vi "main 1.2 dev.vi"() -> ()   [LabVIEW 2015]
uses:
  subvi/PHOIBOS/DEFINITIONS/DEF_dev_state.ctl
  subvi/PHOIBOS/DEFINITIONS/DEF_dev_type.ctl
  <vilib>/Analysis/6fits.llb/Curve Fitting Criteria.ctl
  <vilib>/Analysis/_algsub.llb/Real Vector Norm.vi
  <vilib>/Analysis/1siggen.llb/Ramp Pattern by Samples.vi
  <vilib>/DAQmx/create/channels.llb/DAQmx Create Channel (DI-Digital Input).vi
  <vilib>/Utility/file.llb/Write Delimited Spreadsheet (DBL).vi
  <vilib>/Utility/file.llb/Write Delimited Spreadsheet (string).vi
  <vilib>/Utility/file.llb/Read Delimited Spreadsheet (string).vi
  subvi/Newport ESP301/Newport ESP301.lvlib
  subvi/sp_manip.llb/sp_manip_lib.lvlib
  subvi/sp_manip.llb/tcp_gateway.lvlib
  <vilib>/Analysis/NI_AALBase.lvlib
  <vilib>/Analysis/NI_AALPro.lvlib
  subvi/ZaberTSeries/ZaberTSeries.lvlib
panel:
  out "Pics L":i32=20
  out "Waveform Chart":dbl(graph)
  out "G2 X":cluster{dbl[], "Ramp Pattern":dbl[]}(graph)
  in  "reset every n pics":bool=TRUE
  in  "pics2avg":i32=50
  in  "abort acq.":bool
  out "G2 Y":cluster{dbl[], "Ramp Pattern":dbl[]}(graph)={[0.0, 0.0, 0.0, 0.0, 0.0, 0.0, 0.0, 0.0, 0.0, 0.0, 0.0, 0.0, 0.0, 0.0, 0.0, 0.0, 0.0, 0.0, 0.0, 0.0, 0.0, 0.0, 0.0, 0.0, 0.0, 0.0, 0.0, 0.0, 0.0, 0.0, 0.0, 0.0, 0.0, 0.0, 0.0, 0.0, 0.0, 0.0, 0.0, 0.0, 0.0, 0.0, 0.0, 0.0, 0.0, 0.0, 0.0, 0.0, 0.0, 0.0, 0.0, 0.0, 0.0, 0.0, 0.0, 0.0, 0.0, 0.0, 0.0, 0.0, 0.0, 0.0, 0.0, 0.0, 0.0, 0.0, 0.0, 0.0, 0.0, 0.0, 0.0, 0.0, 0.0, 0.0, 0.0, 0.0, 0.0, 0.0, 0.0, 0.0, 0.0, 0.0, 0.0, 0.0, 0.0, 0.0, 0.0, 0.0, 0.0, 0.0, 0.0, 0.0, 0.0, 0.0, 0.0, 0.0, 0.0, 0.0, 0.0, 0.0, 0.0, 0.0, 0.0, 0.0, 0.0, 0.0, 0.0, 0.0, 0.0, 0.0, 0.0, 0.0, 0.0, 0.0, 0.0, 0.0, 0.0, 0.0, 0.0, 0.0, 0.0, 0.0, 0.0, 0.0, 0.0, 0.0, 0.0, 0.0, 0.0, 0.0, 0.0, 0.0, 0.0, 0.0, 0.0, 0.0, 0.0, 0.0, 0.0, 0.0, 0.0, 0.0, 0.0, 0.0, 0.0, 0.0, 0.0, 0.0, 0.0, 0.0, 0.0, 0.0, 0.0, 0.0, 0.0, 0.0, 0.0, 0.0, 0.0, 0.0, 0.0, 0.0, 0.0, 0.0, 0.0, 0.0, 0.0, 0.0, 0.0, 0.0, 0.0, 0.0, 0.0, 0.0, 0.0, 0.0, 0.0, 0.0, 0.0, 0.0, 0.0, 0.0, 0.0, 0.0, 0.0, 0.0, 0.0, 0.0, 0.0, 0.0, 0.0, 0.0, 0.0, 0.0, 0.0, 0.0, 0.0, 0.0, 0.0, 0.0, 0.0, 0.0, 0.0, 0.0, 0.0, 0.0, 0.0, 0.0, 0.0, 0.0, 0.0, 0.0, 0.0, 0.0, 0.0, 0.0, 0.0, 0.0, 0.0, 0.0, 0.0, 0.0, 0.0, 0.0, 0.0, 0.0, 0.0, 0.0, 0.0, 0.0, 0.0, 0.0, 0.0, 0.0, 0.0, 0.0, 0.0, 0.0, 0.0, 0.0, 0.0, 0.0, 0.0, 0.0, 0.0, 0.0, 0.0, 0.0, 0.0, 0.0, 0.0, 0.0, 0.0, 0.0, 0.0, 0.0], "Ramp Pattern"=[0.0, 1.003921568627451, 2.007843137254902, 3.011764705882353, 4.015686274509804, 5.019607843137255, 6.023529411764706, 7.027450980392157, 8.031372549019608, 9.035294117647059, 10.03921568627451, 11.04313725490196, 12.047058823529412, 13.050980392156863, 14.054901960784314, 15.058823529411764, 16.062745098039215, 17.066666666666666, 18.070588235294117, 19.07450980392157, 20.07843137254902, 21.08235294117647, 22.08627450980392, 23.090196078431372, 24.094117647058823, 25.098039215686274, 26.101960784313725, 27.105882352941176, 28.109803921568627, 29.113725490196078, 30.11764705882353, 31.12156862745098, 32.12549019607843, 33.129411764705885, 34.13333333333333, 35.13725490196079, 36.141176470588235, 37.14509803921569, 38.14901960784314, 39.15294117647059, 40.15686274509804, 41.16078431372549, 42.16470588235294, 43.168627450980395, 44.17254901960784, 45.1764705882353, 46.180392156862744, 47.1843137254902, 48.188235294117646, 49.1921568627451, 50.19607843137255, 51.2, 52.20392156862745, 53.207843137254905, 54.21176470588235, 55.21568627450981, 56.219607843137254, 57.22352941176471, 58.227450980392156, 59.23137254901961, 60.23529411764706, 61.23921568627451, 62.24313725490196, 63.247058823529414, 64.25098039215686, 65.25490196078431, 66.25882352941177, 67.26274509803922, 68.26666666666667, 69.27058823529411, 70.27450980392157, 71.27843137254902, 72.28235294117647, 73.28627450980392, 74.29019607843138, 75.29411764705883, 76.29803921568627, 77.30196078431372, 78.30588235294118, 79.30980392156863, 80.31372549019608, 81.31764705882352, 82.32156862745099, 83.32549019607843, 84.32941176470588, 85.33333333333333, 86.33725490196079, 87.34117647058824, 88.34509803921569, 89.34901960784313, 90.3529411764706, 91.35686274509804, 92.36078431372549, 93.36470588235294, 94.3686274509804, 95.37254901960785, 96.37647058823529, 97.38039215686274, 98.3843137254902, 99.38823529411765, 100.3921568627451, 101.39607843137254, 102.4, 103.40392156862745, 104.4078431372549, 105.41176470588235, 106.41568627450981, 107.41960784313726, 108.4235294117647, 109.42745098039215, 110.43137254901961, 111.43529411764706, 112.43921568627451, 113.44313725490196, 114.44705882352942, 115.45098039215686, 116.45490196078431, 117.45882352941176, 118.46274509803922, 119.46666666666667, 120.47058823529412, 121.47450980392156, 122.47843137254903, 123.48235294117647, 124.48627450980392, 125.49019607843137, 126.49411764705883, 127.49803921568628, 128.50196078431372, 129.50588235294117, 130.50980392156862, 131.51372549019607, 132.51764705882354, 133.521568627451, 134.52549019607844, 135.52941176470588, 136.53333333333333, 137.53725490196078, 138.54117647058823, 139.54509803921567, 140.54901960784315, 141.5529411764706, 142.55686274509804, 143.5607843137255, 144.56470588235294, 145.5686274509804, 146.57254901960783, 147.57647058823528, 148.58039215686276, 149.5843137254902, 150.58823529411765, 151.5921568627451, 152.59607843137255, 153.6, 154.60392156862744, 155.6078431372549, 156.61176470588236, 157.6156862745098, 158.61960784313726, 159.6235294117647, 160.62745098039215, 161.6313725490196, 162.63529411764705, 163.6392156862745, 164.64313725490197, 165.64705882352942, 166.65098039215687, 167.65490196078431, 168.65882352941176, 169.6627450980392, 170.66666666666666, 171.6705882352941, 172.67450980392158, 173.67843137254903, 174.68235294117648, 175.68627450980392, 176.69019607843137, 177.69411764705882, 178.69803921568626, 179.7019607843137, 180.7058823529412, 181.70980392156864, 182.71372549019608, 183.71764705882353, 184.72156862745098, 185.72549019607843, 186.72941176470587, 187.73333333333332, 188.7372549019608, 189.74117647058824, 190.7450980392157, 191.74901960784314, 192.75294117647059, 193.75686274509803, 194.76078431372548, 195.76470588235293, 196.7686274509804, 197.77254901960785, 198.7764705882353, 199.78039215686275, 200.7843137254902, 201.78823529411764, 202.7921568627451, 203.79607843137254, 204.8, 205.80392156862746, 206.8078431372549, 207.81176470588235, 208.8156862745098, 209.81960784313725, 210.8235294117647, 211.82745098039214, 212.83137254901962, 213.83529411764707, 214.8392156862745, 215.84313725490196, 216.8470588235294, 217.85098039215686, 218.8549019607843, 219.85882352941175, 220.86274509803923, 221.86666666666667, 222.87058823529412, 223.87450980392157, 224.87843137254902, 225.88235294117646, 226.8862745098039, 227.89019607843136, 228.89411764705883, 229.89803921568628, 230.90196078431373, 231.90588235294118, 232.90980392156862, 233.91372549019607, 234.91764705882352, 235.92156862745097, 236.92549019607844, 237.9294117647059, 238.93333333333334, 239.93725490196078, 240.94117647058823, 241.94509803921568, 242.94901960784313, 243.95294117647057, 244.95686274509805, 245.9607843137255, 246.96470588235294, 247.9686274509804, 248.97254901960784, 249.9764705882353, 250.98039215686273, 251.98431372549018, 252.98823529411766, 253.9921568627451, 254.99607843137255, 256.0]}
  out "ETA":timestamp=timestamp(3553173084.423481 s since 1904-01-01) format="%<%H:%M:%S>T"
  out "acq. imgs":i32=20
  out "snap_prog":dbl(slide)=1.0 scale=0.0..1.0
  in  "BasePath":path=path "Z:/PESdata"
  in  "cam_liveavg":bool=TRUE caption="live average"
  out "cam_fps":dbl=19.770971874875205 caption="FPS" format="%.1g"
  out "sideimg":dbl[][](graph)
  out "RunNumber":u16=50
  out "sum":dbl format="%#.2g"
  out "max":dbl
  out "mainimg":dbl[][](graph)
  out "ESP_con?":bool=TRUE caption="ESP301"
  out "phoib_con?":bool caption="PHOIBOS"
  out "manip_con?":bool=TRUE caption="manipulator"
  out "cam_con?":bool caption="camera"
  in  "main_close":bool
  in  "Tab Control":enum32{"live", "1D scan", "devices"}(tab)=enum."1D scan"
  in  "mirr_go":bool
  in  "ESP_opent0file":bool
  in  "mirr_rel":i32=20 caption="relative [steps]"
  in  "mirr_Y-":bool
  in  "mirr_Y+":bool
  in  "mirr_X+":bool
  in  "mirr_X-":bool
  in  "manip_deltas":dbl[](array[numeric])=[0.0, 0.0, 5.0, 0.0, 0.0, 0.0] caption="delta" format="%#.5g"
  in  "aq.mode":enum32{"Radio Selection 1", "Radio Selection 2"}(radio)=enum."Radio Selection 2"
  in  "dark avg":i32=100
  in  "cam_avgs":i32=20 caption="N"
  in  "ESP_delta":dbl caption="relative [mm]"
  in  "ESP_-":bool
  in  "ESP_+":bool
  in  "ESP_go":bool
  in  "ESP_dest_t":dbl=-12656.75602819869 caption="[fs]"
  in  "ESP_dest":dbl=25.0 caption="[mm]"
  in  "ESP_set_t0":bool
  in  "phoib_I_6s":dbl=3200.0
  in  "phoib_I_5s":dbl=1500.0
  in  "phoib_I_4s":dbl=4.558
  in  "phoib_I_3s":dbl=-7.0
  in  "phoib_I_2s":dbl=30.0
  in  "phoib_I_1s":dbl=18.0
  in  "phoib_standby":bool
  in  "phoib_set":bool
  out "phoib_I_6":dbl caption="Screen Voltage"
  out "phoib_I_5":dbl caption="Detctor Voltage"
  out "phoib_I_4":dbl caption="Work Function"
  out "phoib_I_3":dbl caption="Coil Current"
  out "phoib_I_2":dbl caption="Pass Energy"
  out "phoib_I_1":dbl caption="Kinetic Energy"
  out "Saved Positions":string[][](table)=[["ertwertwert", "-2.299945", "-2.030214", "38.900024", "50.000762", "0.000887", "-97.998082"], ["uztgugt", "-14.999451", "-13.638894", "442.380066", "13.998380", "-1.893758", "-76.305838"], ["asdf", "-14.999451", "-13.638894", "442.380066", "13.998380", "-1.893758", "-76.305838"], ["test3", "-14.999451", "-13.638894", "441.380066", "13.998380", "-1.893758", "-76.305838"]]
  in  "Save Pos":bool
  in  "Load":bool
  in  "Delete":bool
  in  "ManipRel +":bool
  in  "ManipRel -":bool
  in  "Move Abs":bool
  in  "stop manip":bool
  in  "dest":dbl[](array[numeric])=[-2.599774415331921, 2.6001372083008483, 64.7374267578125, 44.999124169862, 0.0008789063100814859, -80.99718876558107] caption="destination" format="%#.5g"
  out "axis":string[](array[string])=["x", "y", "z", "polar", "tilt", "azimut"]
  out "pos":dbl[](array[numeric])=[-1.8981328134268227, 1.9037561044451934, 84.7381591796875, 38.14189713860625, 0.0008789063100814859, -70.9987511093555] caption="position" format="%.5f"
  in  "ana_mode":T1(ring)=enum."WideAngleMode"
  in  "ana_voltrange":enum16{"3.5kV", "1.5kV", "400V", "100V", "10V"}(ring)=enum."400V"
  out "ESP_pos":dbl=31.74535 caption="Position"
  out "ESP_delay":dbl=45000.131390897084 caption="Delay"
  out "ESP_t0":dbl=25.0 caption="Time Zero @"
  out "phoib_I_7":dbl caption="Conversion Voltage"
  in  "phoib_I_7s":dbl=-26.0
  in  "phoib_I_8s":dbl=0.0039
  in  "phoib_I_9s":dbl=0.0039
  out "phoib_I_8":dbl caption="FD1"
  out "phoib_I_9":dbl caption="FD2"
  in  "gain":bool
  in  "cam_exp":u32=50 caption="exposure [ms]"
  in  "binning":u16(ring)=2 items=["X 1", "X 2", "X 4", "X 8"]
  in  "cam_dark?":bool=TRUE caption="subtract dark?"
  in  "cam_dark":bool
  in  "cam_saveimg":bool
  in  "e-size":u8
  in  "lower threshold":i32=50
  in  "count?":bool
  in  "ROI Left":i32=1
  in  "ROI Right":i32=43
  in  "ROI Top":i32=1
  in  "ROI Bottom":i32=33
  out "moving?":bool[](array[boolean])
  out "mirr_posX":i32=-9907 caption="X"
  out "mirr_posY":i32=-7260 caption="Y"
  in  "mirr_dest":i32[](array[numeric])=[-64, -2601]
  in  "gauss fit":bool
  out "anglegraph":dbl[][](graph)
  out "intensitygraph":T2(graph)
  in  "scan_selector":enum32{"delay", "manip", "mirror", "volt"}(tab)=enum."mirror"
  in  "scan_manip_setstart":bool
  in  "scan_manip_start":dbl[](array[numeric])=[-2.6172862113166087, -0.009888298846365134, 68.5008544921875, -46.363686276590336, 11.108982061941884, -218.56360350415366] caption="start position" format="%#.5g"
  in  "scan_manip_deltas":dbl[](array[numeric])=[0.0, 0.0, 0.0, 0.0, 10.0, 0.0] caption="direction vector\n(gets normed)" format="%#.5g"
  in  "scan_mirr_start":i32[](array[numeric])=[-64, -2601]
  in  "scan_mirr_deltas":i32[](array[numeric])=[0, 0] caption="direction vector\n(gets normed)"
  in  "scan_mirr_setstart":bool
  in  "scan_volt_parameter":string(combo)="Kinetic Energy"
  in  "meas_iter":i32=60 caption="Iterations"
  out "duration [HH:MM:SS]":dbl=4512.494100093842 format="%<%H:%M:%S>t"
  out "disk [MB]":dbl=1028.5800000000002
  out "RAM [MB]":dbl=17.143
  out "total steps":i32=1860
  out "measpoints":i32=31
  in  "load delay table":bool
  in  "scan_go":bool
  in  "waypoints":string[][](table)=[["-100000", "5000"], ["50000", ""], ["", ""]]
  in  "stop after step":bool
  out "scan":dbl(slide)=0.967741935483871 scale=0.0..1.0
  out "iteration":dbl(slide)=0.03333333333333333 scale=0.0..1.0
  out "current scan":i32=30
  out "current iteration":i32=2
  in  "time/step [s]":dbl=2.426072096824646
  in  "stop after iteration":bool
  out "energygraph":dbl[][](graph)
  out "center":dbl
  in  "mirr_init":bool
  in  "mirr_release":bool
  in  "mirr_Y#":u8=2
  in  "manip_init":bool
  in  "manip_release":bool
  in  "phoib_init":bool
  in  "phoib_release":bool
  in  "ESP_init":bool
  in  "ESP_release":bool
  in  "ESP301 VISA":refnum<visa-resource-name>="COM8"
  in  "board number":i32
  in  "cam_init":bool
  in  "cam_release":bool
  out "cam_error":errorcluster
  out "phoib_error":errorcluster
  out "state":T3 items=["Off"=-1, "Standby"=0, "On"=1]
  in  "ESP Axis":i32=1 min=1 max=3
  out "error out":errorcluster
  out "error out 2":errorcluster
  out "mirr_Error":errorcluster
  in  "mirr_VISA":refnum<visa-resource-name>="COM7"
  in  "mirr_X#":u8=1
  in  "Operating mode\nHP & QE / HS & DiCam Pro":u32=1
  in  "Frame trigger \n(High Performance and QE only)":u16
  # "camera"
  # "analyzer"
  # "manipulator"
  # "aquisition"
  # "delay stage"
  # "mirror"
  # "Position"
  # "Destination"
  # "- no settings -"
  # "waypoints are absolute values"
  # "X\nY\nZ\npolar\ntilt\nazimut"
  # "waypoint \"0\" is start position"
  # "X\nY"
  # "waypoint \"0\" is start position"
  # "waypoints are absolute values"
  # "camera"
  # "phoibos"
  # "ESP301"
  # "manipulator"
  # "mirror"
  # "0 = sequential\n1 = simultaneous"
  # "0 = internal\n1 = external rising\n2 = external falling"
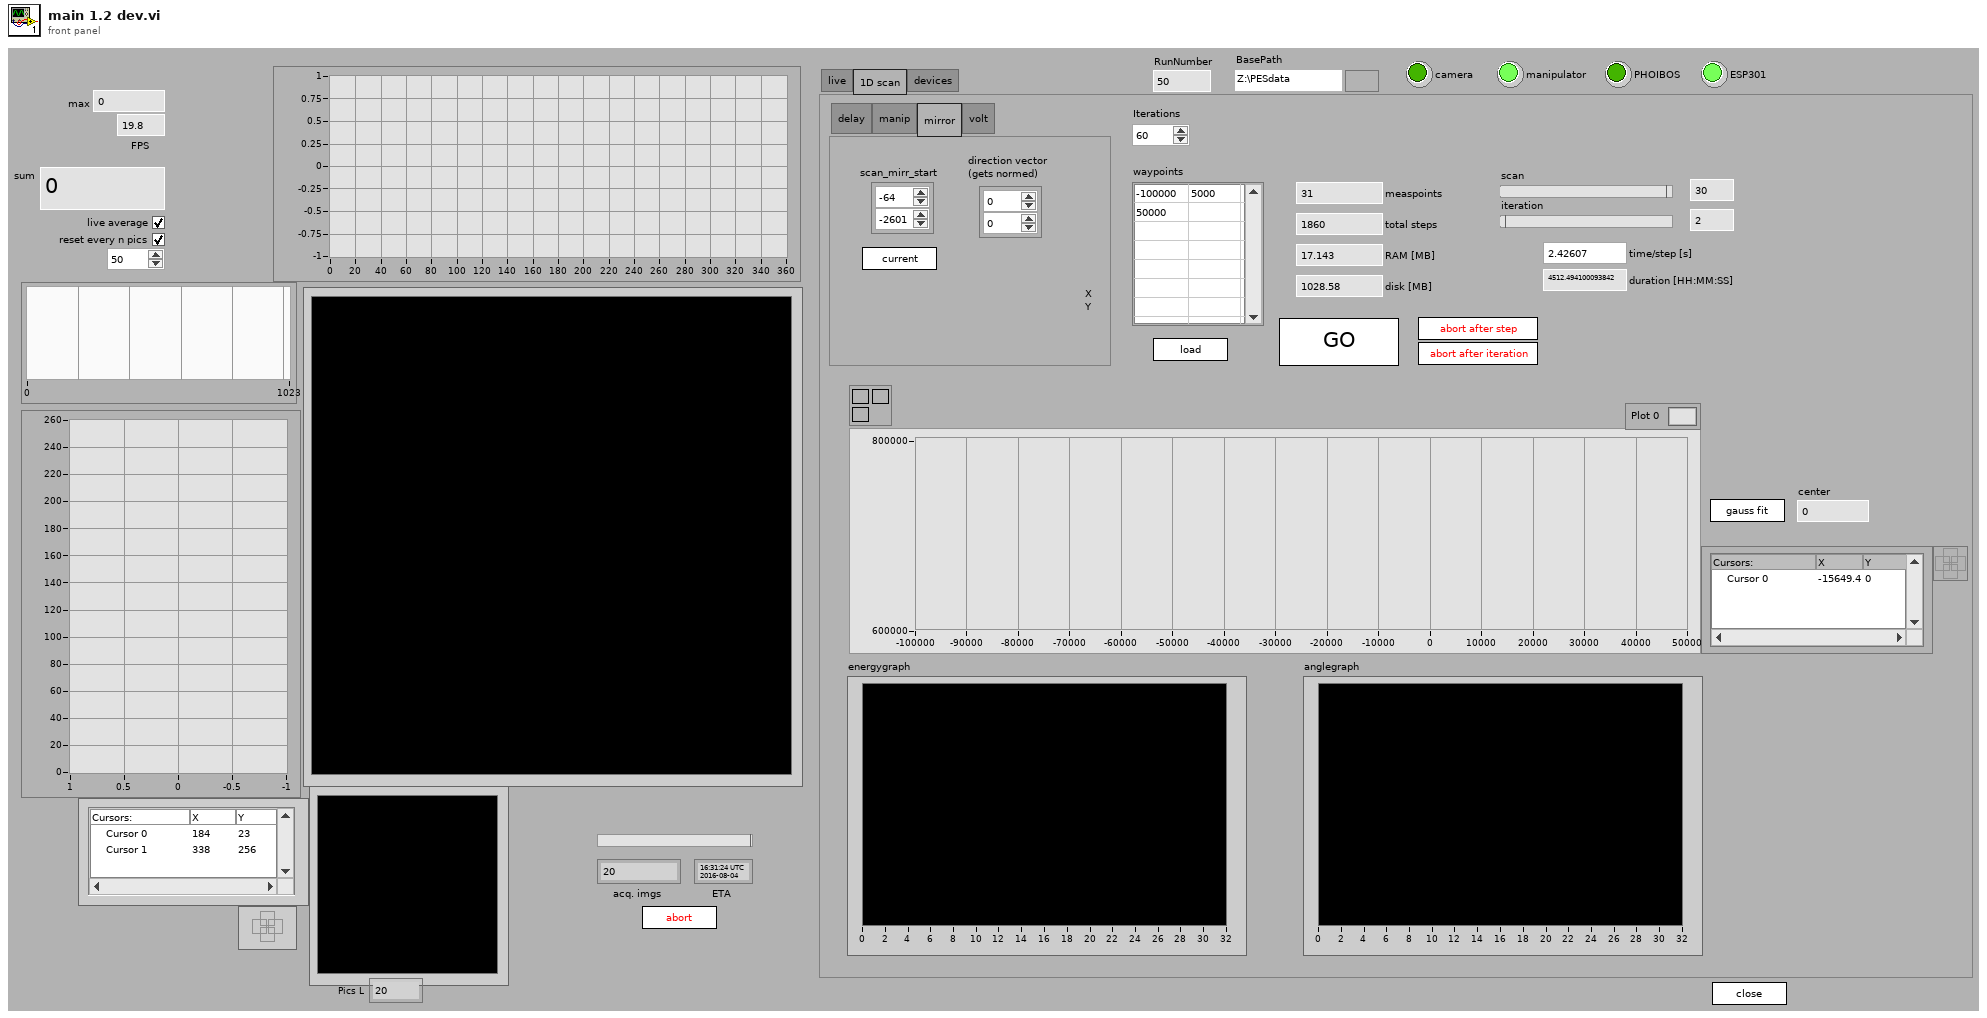
[diagram p1: front panel]
types:
  T1 = enum16{"HighMagnification", "MediumMagnification", "LowMagnification", "HighAngularDispersion", "MediumAngularDispersion", "LowAngularDispersion", "WideAngleMode", "LargeArea", "MediumArea", "SmallArea", "HighMagnification2", "SmallArea2", "ImagingMode"}
  T2 = cluster{"Array":dbl[], "Intensity Chart":dbl[]}[]
  T3 = typedef "DEF_dev_state.ctl" = i32
  T4 = cluster{"queue out":refnum<queue>, "queue out":refnum<queue>, "queue out":refnum<queue>, "queue out":refnum<queue>, "queue out":refnum<queue>}
  T5 = typedef "LVCursorListTypeDef.ctl" = cluster{"Name":string, "Color":u32, "Style":u8, "Point Style":u8, "Name Visible":bool, "Allow Drag":bool, "Cursor Mode":u32, "Plot":i32, "Index":i32, "Position":cluster{"X":dbl, "Y":dbl}, "X Scale":u32, "Y Scale":u32, "Watch Plots":i32[], "Watch All Plots":bool, "Plot Area":i32, "Label Offset":cluster{"X":dbl, "Y":dbl}}[]
  T6 = typedef "NI_AALPro.lvlib/Curve Fitting Criteria.ctl" = u16
  T7 = cluster{"Array":dbl[], "Best Gaussian Fit":dbl[]}
  T8 = cluster{"Array":dbl[], "Best Gaussian Fit":dbl[]}[]
  T9 = cluster{"Camera type":u32, "Operating mode\nHP & QE / HS & DiCam Pro ":u32, "Frame trigger \n(High Performance and QE only)":u16, "Sequence trigger":u16, "Low Light\n(QE only)":bool, "Gain":bool, "Horzontal\nbinning":u16, "Vertical\nbinning ":u16, "ROI Left":i32, "ROI Right":i32, "ROI Top":i32, "ROI Bottom":i32}
  T10 = cluster{"Name":string, "Color":u32, "Style":u8, "Point Style":u8, "Name Visible":bool, "Allow Drag":bool, "Cursor Mode":u32, "Plot":i32, "Index":i32, "Position":cluster{"X":dbl, "Y":dbl}, "X Scale":u32, "Y Scale":u32, "Watch Plots":i32[], "Watch All Plots":bool, "Plot Area":i32, "Label Offset":cluster{"X":dbl, "Y":dbl}}
  T11 = cluster{"mirr_X#":u8, "Command":u8, dbl, "Response Count":i32}
  T12 = cluster{"mirr_Y#":u8, "Command":u8, dbl, "Response Count":i32}
  T13 = cluster{i32, "Command":u8, i32, "Response Count":i32}
  T14 = cluster{"Axis_Name":string, "Axis_Type":string, "Axis_Position":dbl, "continous":bool, "moving":bool}[]
  T15 = typedef "DEF_dev_type.ctl" = enum32{"devA (analyzer)", "devD (detector)"}
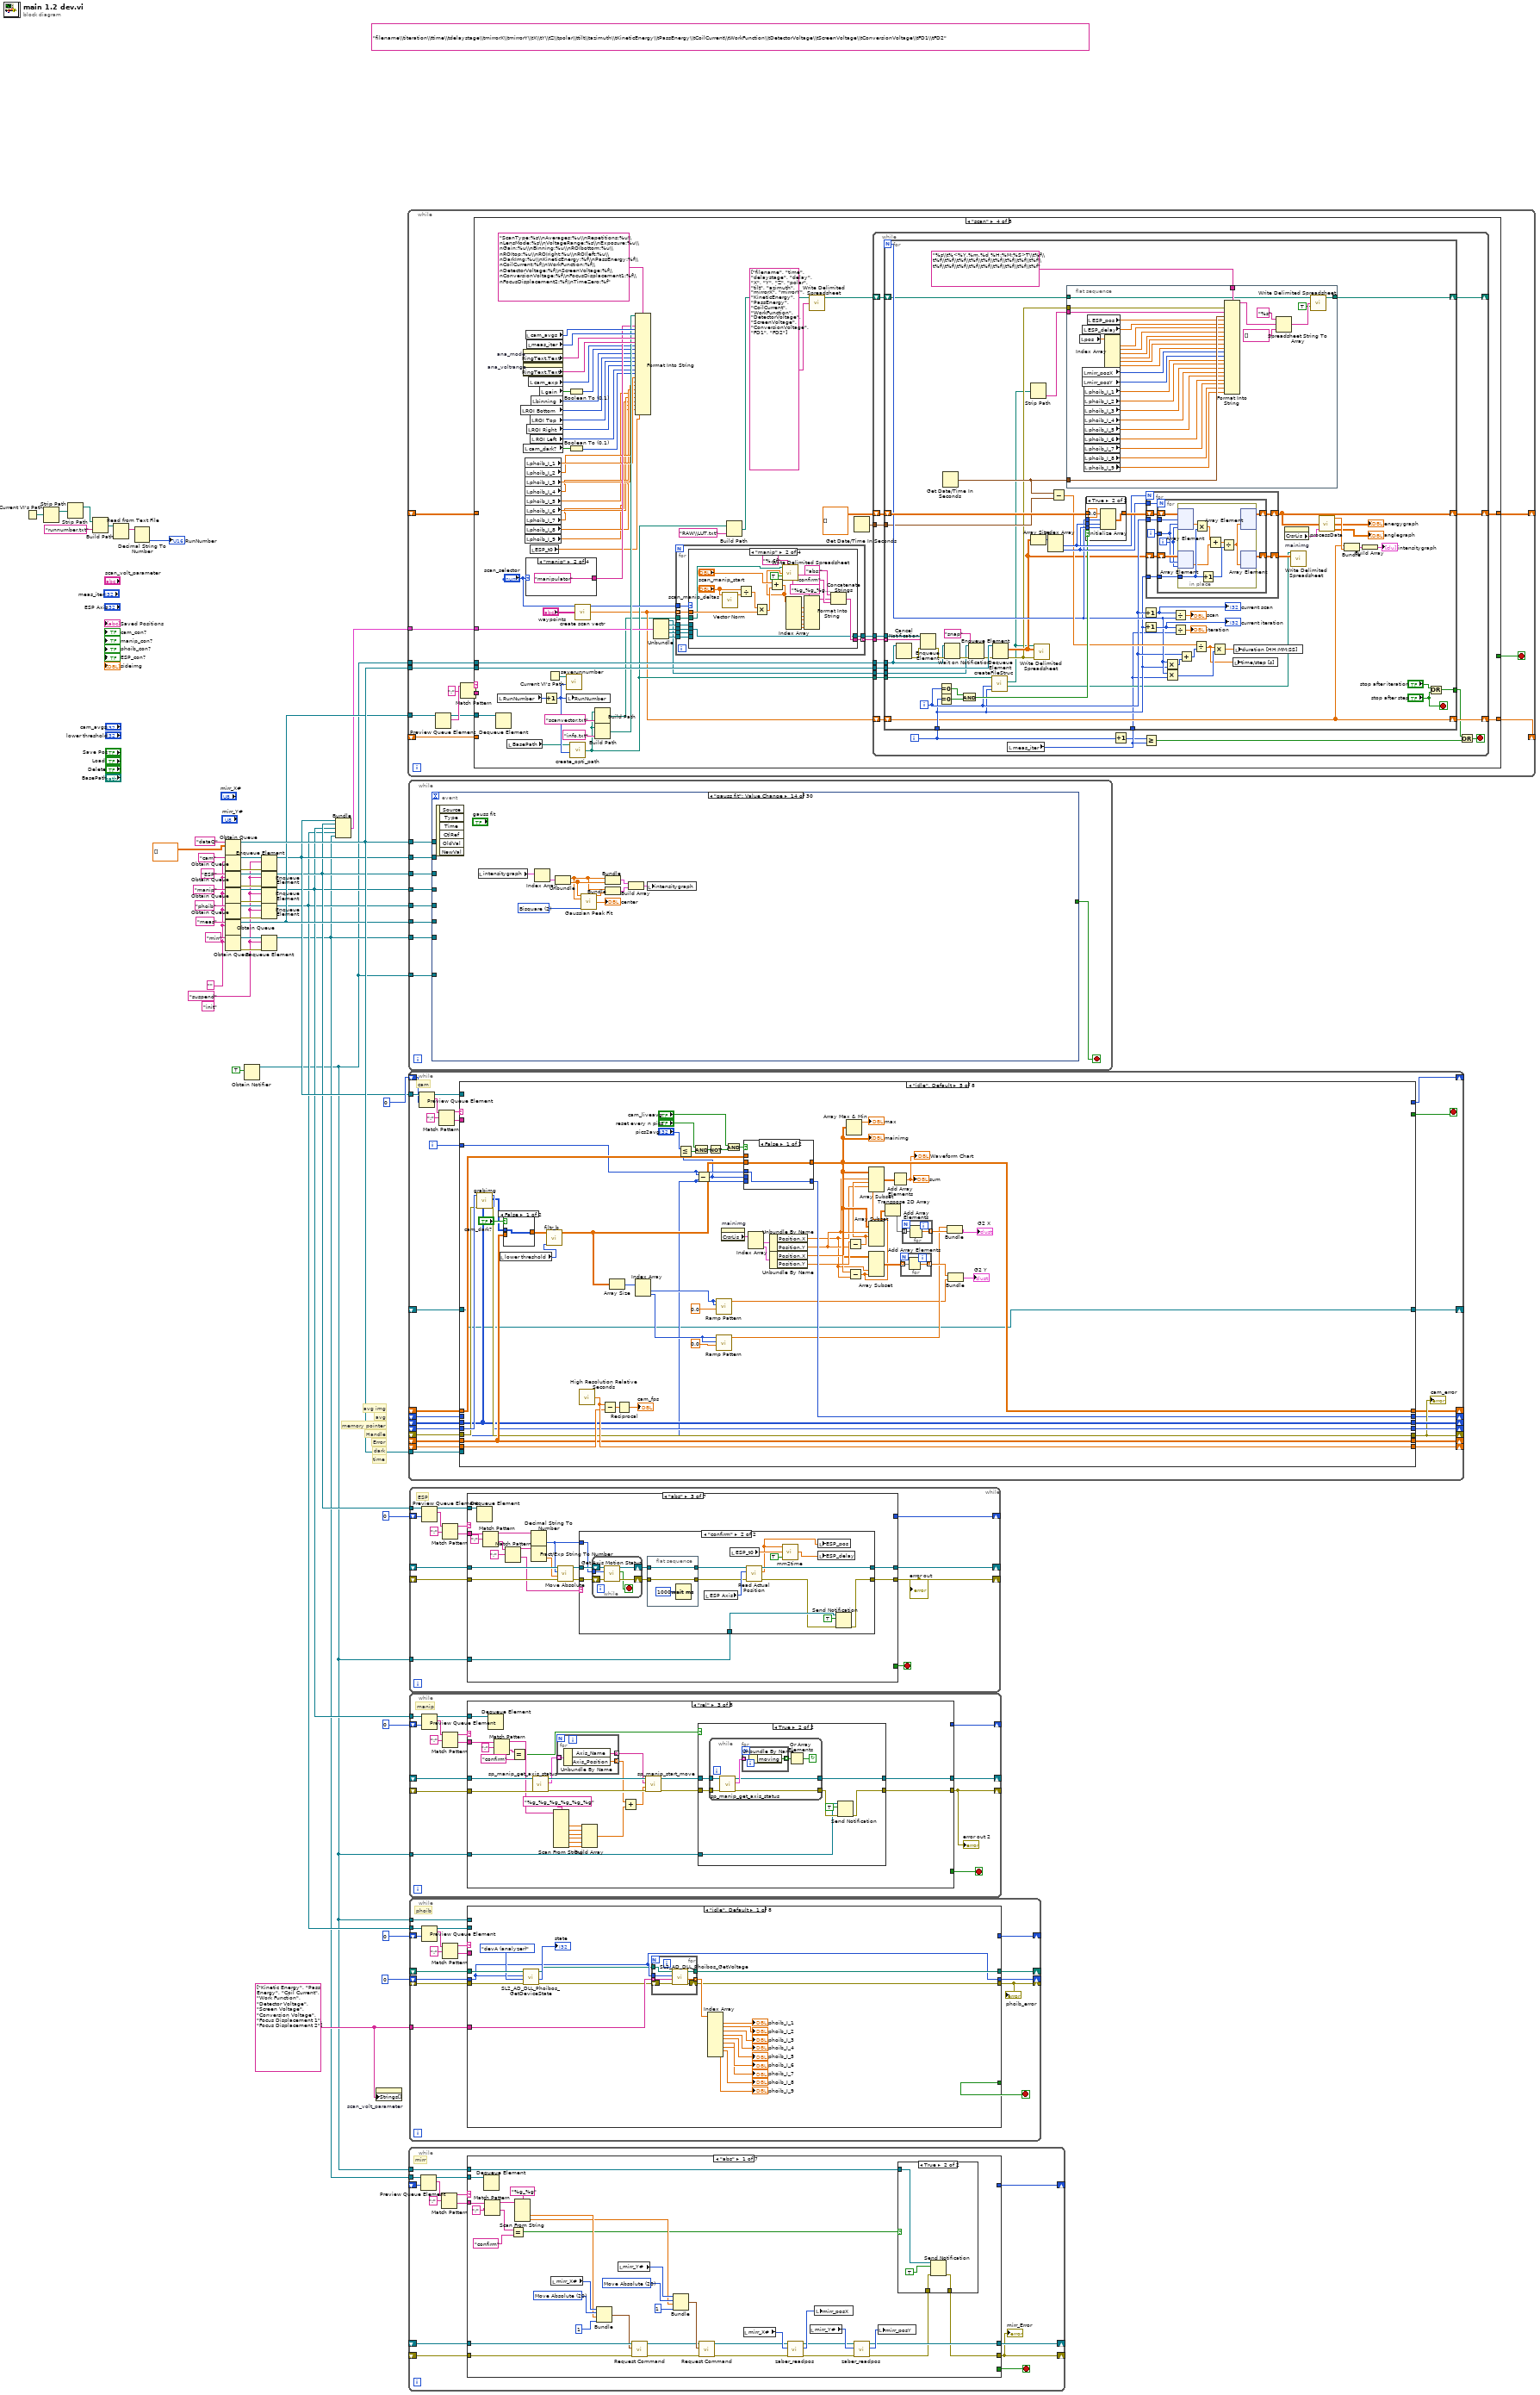
[diagram p0: block diagram]
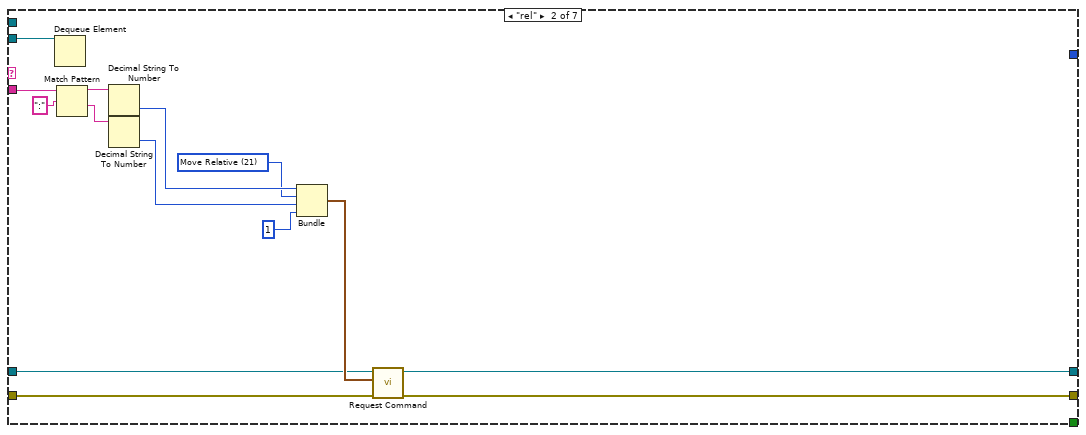
[diagram p3: hidden frame]
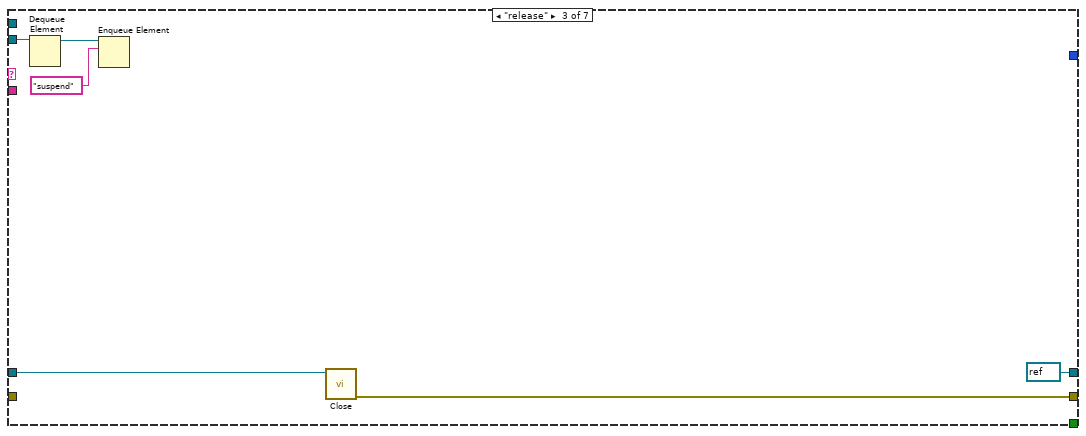
[diagram p4: hidden frame]
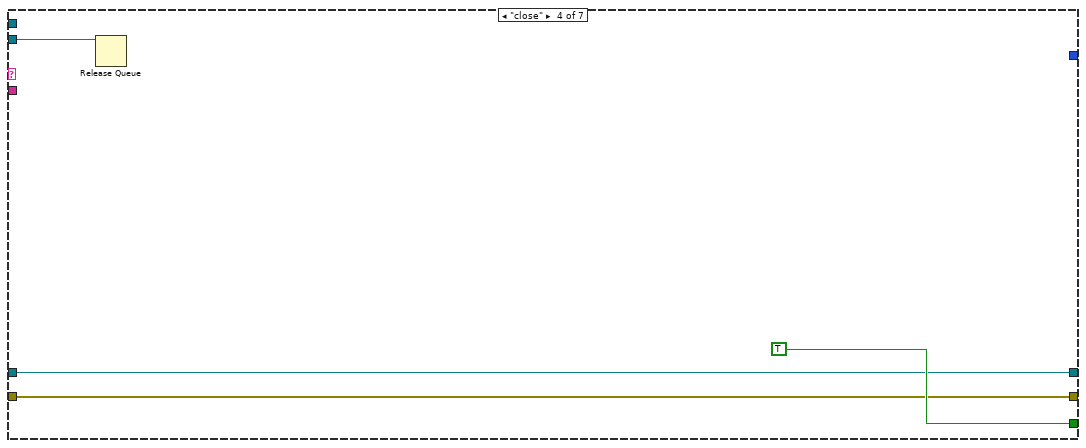
[diagram p5: hidden frame]
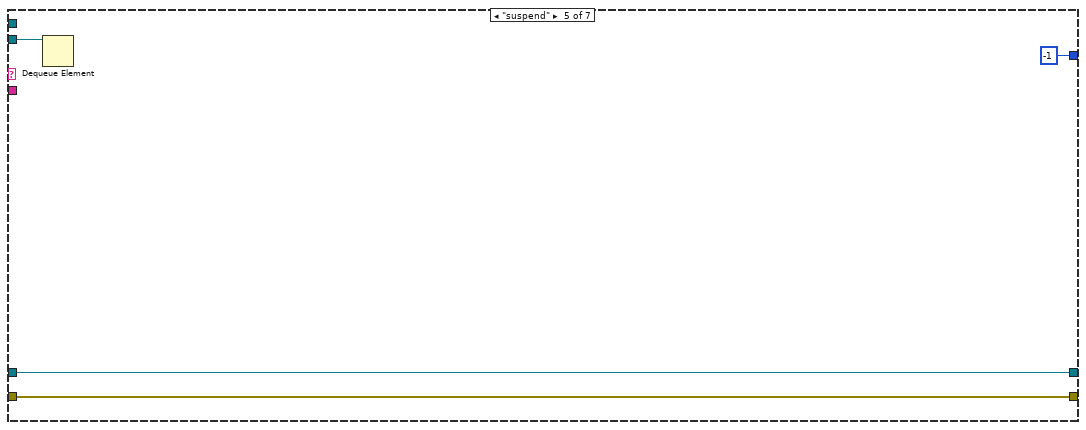
[diagram p6: hidden frame]
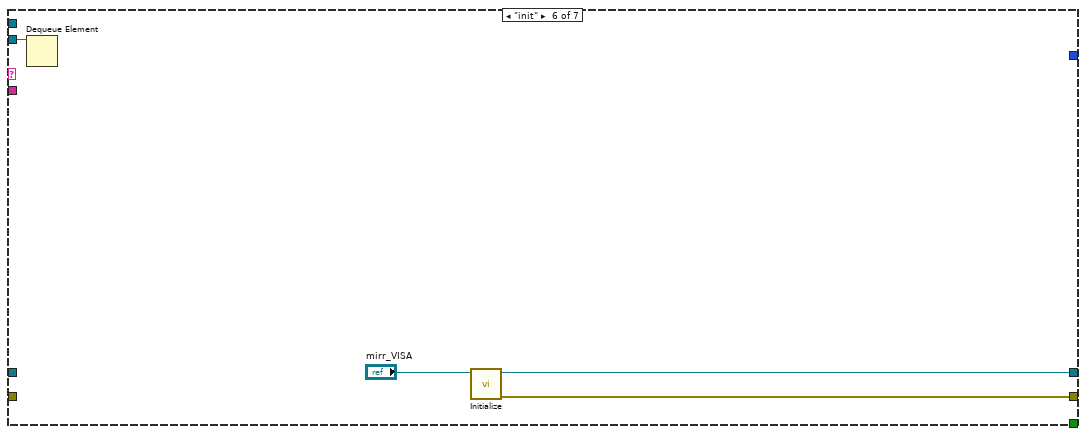
[diagram p7: hidden frame]
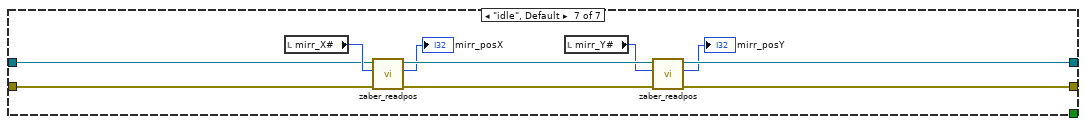
[diagram p8: hidden frame]
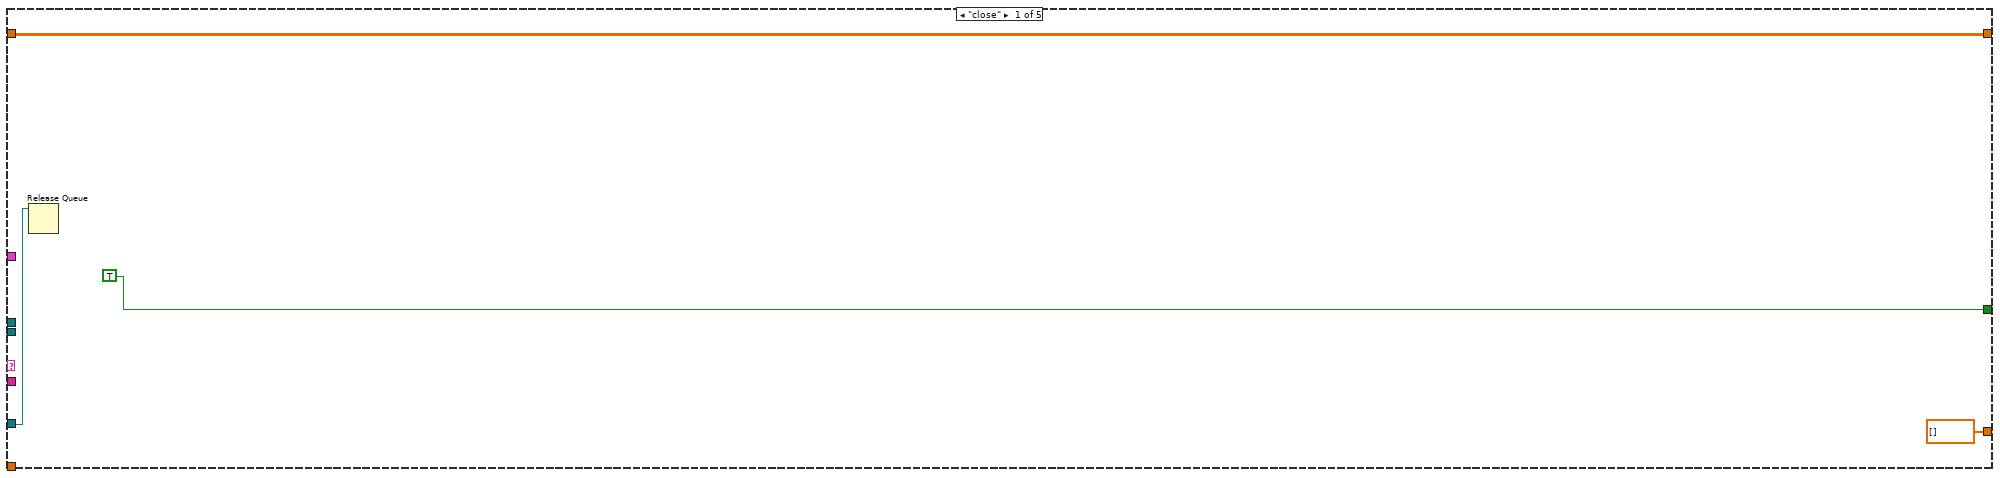
[diagram p9: hidden frame]
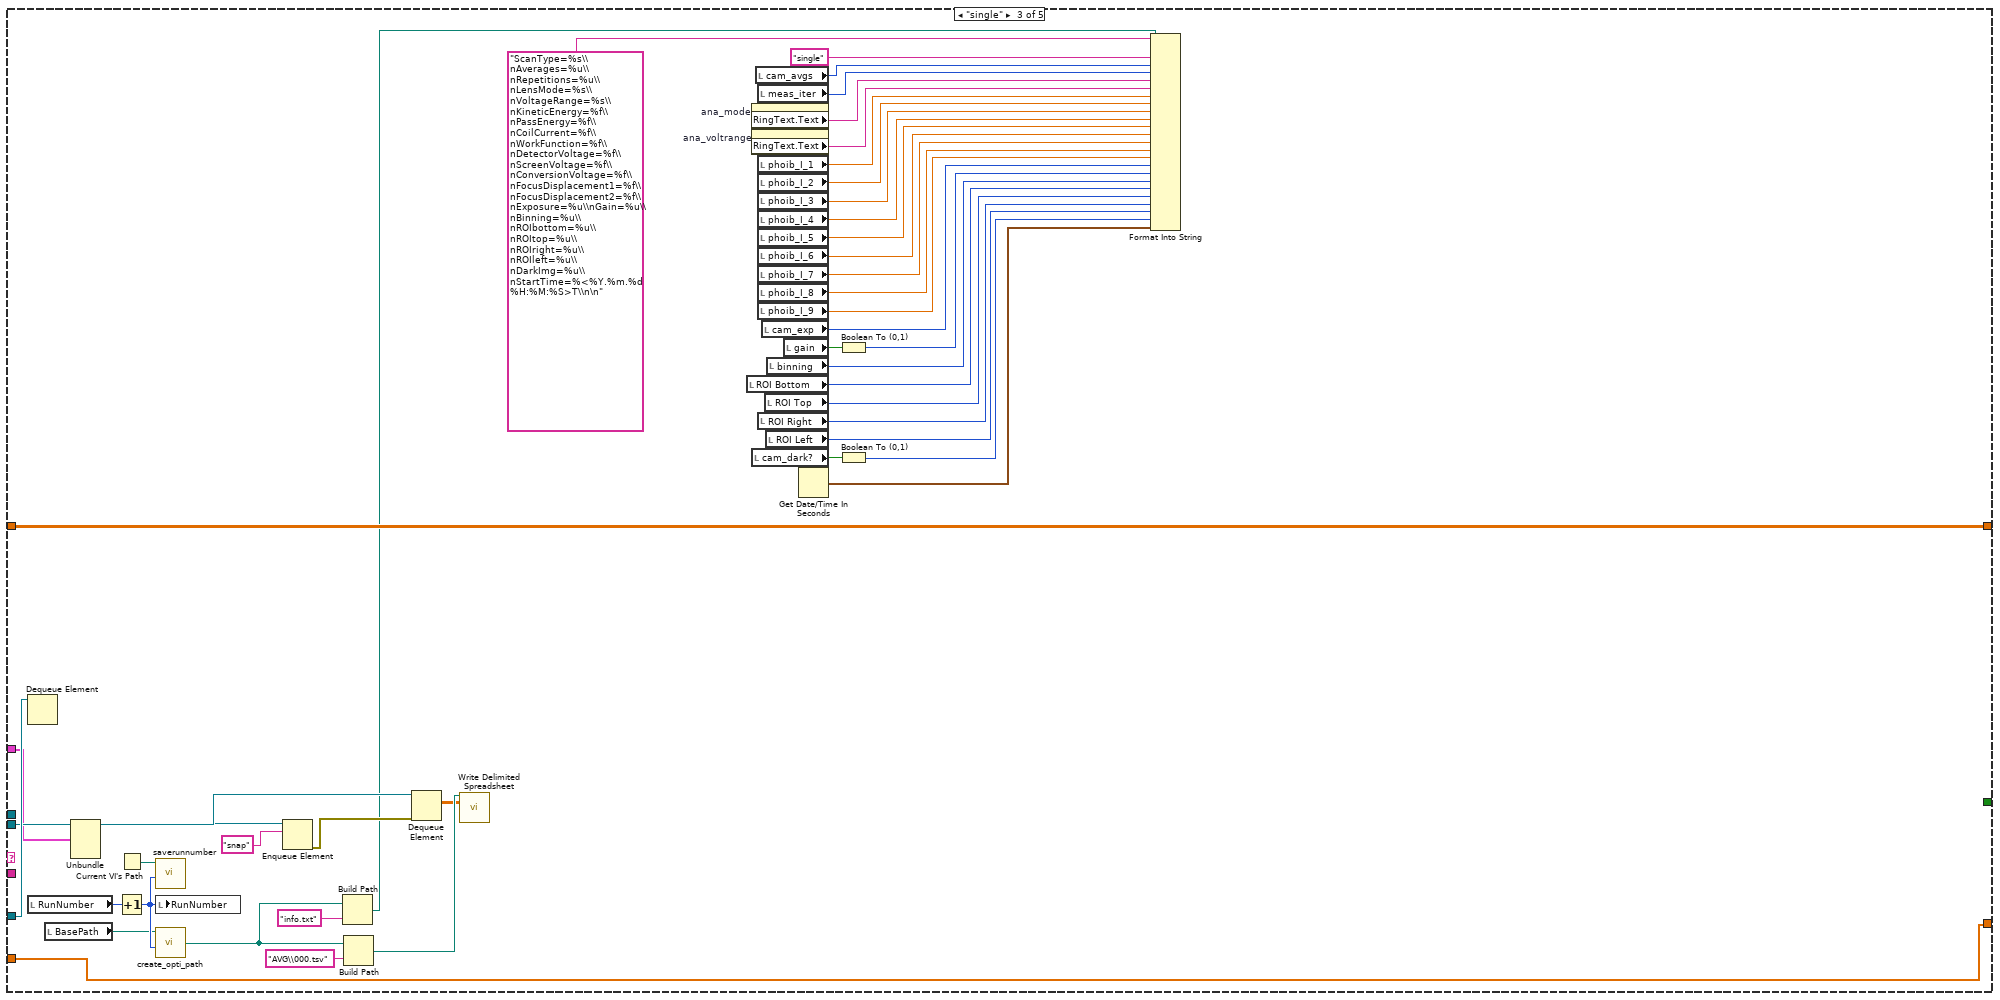
[diagram p11: hidden frame]
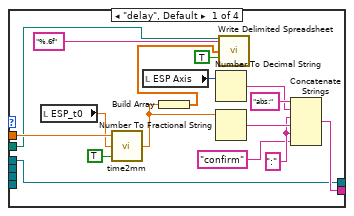
[diagram p13: hidden frame]
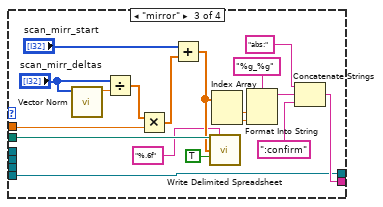
[diagram p14: hidden frame]
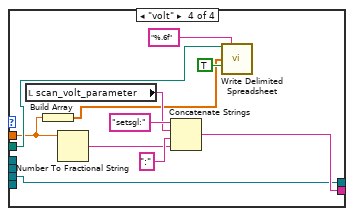
[diagram p15: hidden frame]
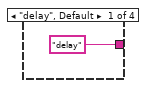
[diagram p16: hidden frame]
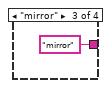
[diagram p17: hidden frame]
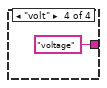
[diagram p18: hidden frame]
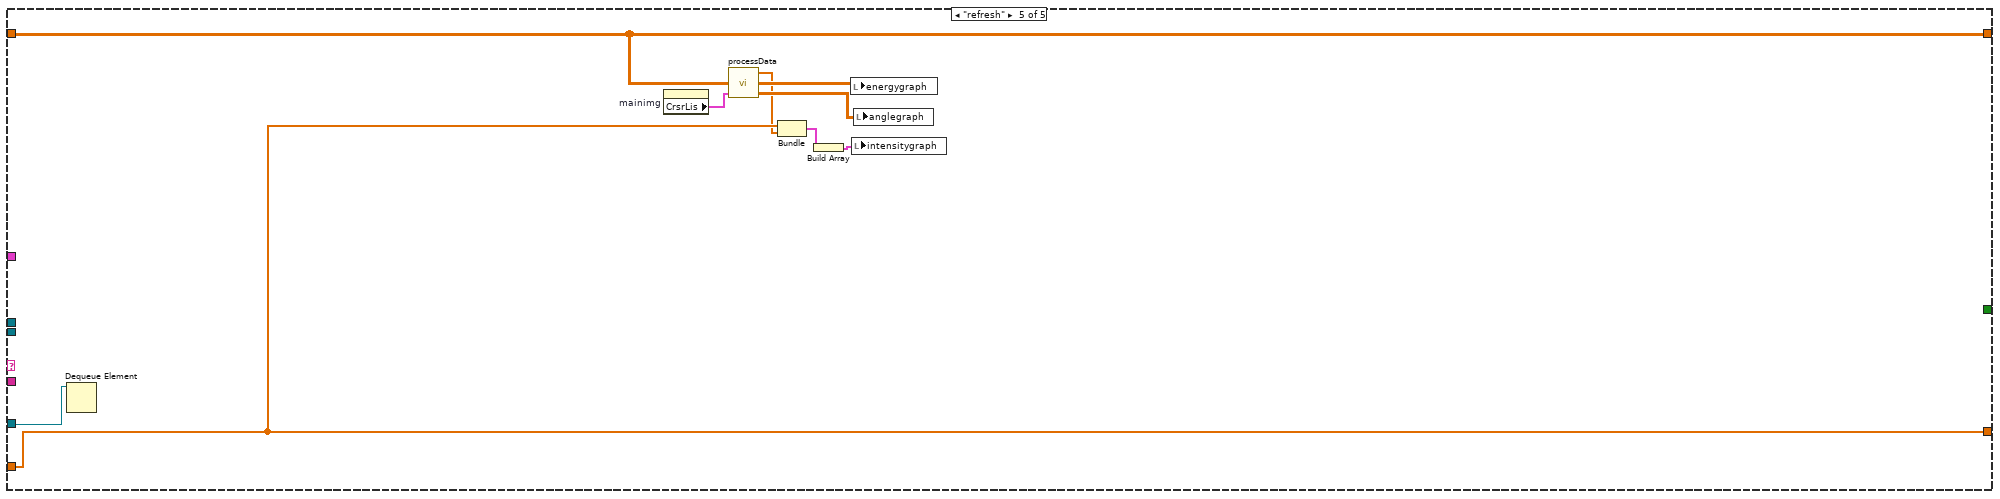
[diagram p19: hidden frame]
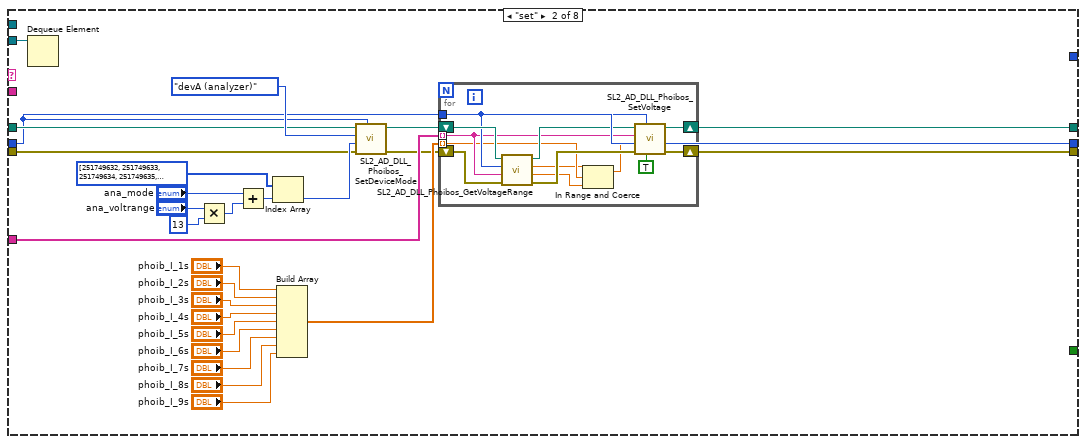
[diagram p20: hidden frame]
diagram:
  (unwired) "filename\\titeration\\ttime\\tdelaystage\\tmirrorX\\tmirrorY\\tX\\tY\\tZ\\tpolar\\ttilt\\tazimuth\\tKineticEnergy\\tPassEnergy\\tCoilCurrent\\tWorkFunction\\tDetectorVoltage\\tScreenVoltage\\tConversionVoltage\\tFD1\\tFD2"
  w9 = string[] ["Kinetic Energy", "Pass Energy", "Coil Current", "Work Function", "Detector Voltage", "Screen Voltage", "Conversion Voltage", "Focus Displacement 1", "Focus Displacement 2"]
  (unwired) "init" ("name (unnamed)")
  w1 = "suspend" ("name (unnamed)")
  w2 = "" ("name (unnamed)")
  # "avg img"
  # "avg"
  # "time"
  # "dark"
  # "Error"
  # "Handle"
  # "memory pointer"
  n1 = Current VI's Path() -> (path=w17:path)
  n2 = Strip Path(path=w17) -> (stripped path=w21:path)  [unwired: 1 out]
  n3 = Strip Path(path=w21) -> (stripped path=w22:path)  [unwired: 1 out]
  n4 = Build Path(base path=w22, name or relative path="runnumber.txt") -> (appended path=w19:path)
  n5 = Read from Text File(file (use dialog)=w19) -> (text=w20:string)  [unwired: 3 in, 3 out]
  n6 = Decimal String To Number(string=w20) -> (number=→"RunNumber":i32)  [unwired: 2 in, 1 out]
  n7 = Obtain Queue(name (unnamed)="dataQ", element data type=dbl[][] []) -> (queue out=w23:refnum<queue>)  [unwired: 3 in, 2 out]
  n8 = Obtain Queue(name (unnamed)="cam", element data type=w2) -> (queue out=w42:refnum<queue>, error out=w41:errorcluster)  [unwired: 3 in, 1 out]
  n9 = Obtain Queue(name (unnamed)="ESP", element data type=w2) -> (queue out=w39:refnum<queue>, error out=w40:errorcluster)  [unwired: 3 in, 1 out]
  n10 = Obtain Queue(name (unnamed)="manip", element data type=w2) -> (queue out=w36:refnum<queue>, error out=w35:errorcluster)  [unwired: 3 in, 1 out]
  n11 = Obtain Queue(name (unnamed)="phoib", element data type=w2) -> (queue out=w33:refnum<queue>, error out=w34:errorcluster)  [unwired: 3 in, 1 out]
  n12 = Obtain Queue(name (unnamed)="meas", element data type=w2) -> (queue out=w16:refnum<queue>)  [unwired: 3 in, 2 out]
  n13 = Obtain Queue(name (unnamed)="mirr", element data type=w2) -> (queue out=w7:refnum<queue>, error out=w6:errorcluster)  [unwired: 3 in, 1 out]
  n14 = Obtain Notifier(notification data type=TRUE) -> (notifier out=w3:refnum<notifier>)  [unwired: 3 in, 2 out]
  n15 = Enqueue Element(queue=w42, element=w1, error in (no error)=w41) -> (queue out=w14:refnum<queue>)  [unwired: 1 in, 2 out]
  n16 = Enqueue Element(queue=w39, element=w1, error in (no error)=w40) -> (queue out=w13:refnum<queue>)  [unwired: 1 in, 2 out]
  n17 = Enqueue Element(queue=w36, element=w1, error in (no error)=w35) -> (queue out=w12:refnum<queue>)  [unwired: 1 in, 2 out]
  n18 = Enqueue Element(queue=w33, element=w1, error in (no error)=w34) -> (queue out=w11:refnum<queue>)  [unwired: 1 in, 2 out]
  n19 = Enqueue Element(queue=w7, element=w1, error in (no error)=w6) -> (queue out=w4:refnum<queue>)  [unwired: 1 in, 2 out]
  n20 = Bundle("queue out"=w14, "queue out"=w13, "queue out"=w12, "queue out"=w11, "queue out"=w4) -> (w15:T4)  [unwired: 1 in]
  n21 = property on="scan_volt_parameter" class="CmbBox"("Strings[]"=w9) -> ()  [unwired: 2 in, 2 out]
  n22 = while {
    tunnel: w23 -> [w57]
    tunnel: w16 -> [w54]
    tunnel: w15 -> [w50]
    shift-right: [w48] -> _
    shift-left: _ -> [w47]
    tunnel: w3 -> [w46]
    shift-right: [w45] -> _
    shift-left: _ -> [w44]
    stop <- w49 stop-if-true
    n23 = Preview Queue Element(queue=w54) -> (queue out=w51:refnum<queue>, element=w56:string)  [unwired: 2 in, 2 out]
    n24 = Match Pattern(string=w56, regular expression=":") -> (before substring=w53:string, after substring=w52:string)  [unwired: 1 in, 2 out]
    n25 = case shown="\"scan\"" w53 {
      tunnel: w57 -> [_ _ w106 w158 _]
      tunnel: w52 -> [_ _ _ _ _]
      tunnel: w51 -> [w61 _ w107 w154 w381]
      tunnel: [TRUE _ _ _ _] -> w49
      tunnel: w50 -> [_ _ w94 w134 _]
      tunnel: [w59 w63 w92 w156 w386] -> w48
      tunnel: w47 -> [w59 w63 w92 _ w386]
      tunnel: w46 -> [_ _ _ w155 _]
      tunnel: [dbl[] [] ("Array") w62 w64 w120 w383] -> w45
      tunnel: w44 -> [_ w62 w64 _ w383]
      frame "close" {
        n26 = Release Queue(queue=w61) -> ()  [unwired: 2 in, 3 out]
      }
      frame "idle", Default {
      }
      frame "single" {
        n27 = Dequeue Element(queue=w107) -> ()  [unwired: 2 in, 4 out]
        n28 = local read "RunNumber"() -> (w101:u16)
        n29 = local read "BasePath"() -> (w102:path)
        n30 = Unbundle(w94) -> ("queue out"=w93:refnum<queue>)  [unwired: 4 out]
        n31 = Increment(x=w101) -> (x+1=w103:u16)
        n32 = Current VI's Path() -> (path=w100:path)
        n33 = call "saverunnumber.vi"("RunNumber"=w103, "VI path"=w100) -> ()  [unwired: 10 in]
        n34 = local write "RunNumber"(w103) -> ()
        n35 = call "create_opti_path.vi"("RunNumber"=w103, "base path"=w102) -> ("Path"=w96:path)  [unwired: 2 in]
        n36 = Enqueue Element(queue=w93, element="snap" ("string")) -> (error out=w104:errorcluster)  [unwired: 2 in, 2 out]
        n37 = Build Path(base path=w96, name or relative path="info.txt") -> (appended path=w65:path)
        n38 = Build Path(base path=w96, name or relative path="AVG\\000.tsv") -> (appended path=w98:path)
        n39 = Dequeue Element(queue=w106, error in (no error)=w104) -> (element=w95:dbl[][])  [unwired: 1 in, 3 out]
        n40 = call-poly <vilib>:"Write Delimited Spreadsheet.vi"("file path (dialog if empty)"=w98, "2D data"=w95) -> ()  [unwired: 12 in, 2 out]
        n41 = local read "ROI Bottom"() -> (w72:i32)
        n42 = property on="ana_mode" class="Enum (strict)"() -> ("RingText.Text"=w87:string)  [unwired: 2 in, 2 out]
        n43 = property on="ana_voltrange" class="Enum (strict)"() -> ("RingText.Text"=w86:string)  [unwired: 2 in, 2 out]
        n44 = local read "cam_dark?"() -> (w68:bool)
        n45 = local read "cam_avgs"() -> (w89:i32)
        n46 = local read "meas_iter"() -> (w88:i32)
        n47 = local read "phoib_I_1"() -> (w85:dbl)
        n48 = local read "phoib_I_2"() -> (w84:dbl)
        n49 = local read "phoib_I_3"() -> (w83:dbl)
        n50 = local read "phoib_I_4"() -> (w82:dbl)
        n51 = local read "phoib_I_5"() -> (w81:dbl)
        n52 = local read "phoib_I_6"() -> (w80:dbl)
        n53 = local read "phoib_I_7"() -> (w79:dbl)
        n54 = local read "phoib_I_8"() -> (w78:dbl)
        n55 = local read "phoib_I_9"() -> (w77:dbl)
        n56 = local read "ROI Right"() -> (w70:i32)
        n57 = local read "cam_exp"() -> (w76:u32)
        n58 = local read "ROI Top"() -> (w71:i32)
        n59 = local read "ROI Left"() -> (w69:i32)
        n60 = local read "binning"() -> (w73:u16)
        n61 = local read "gain"() -> (w75:bool)
        n62 = Get Date/Time In Seconds() -> (seconds since 1Jan1904=w66:timestamp)
        n63 = Boolean To (0,1)(Boolean=w75) -> (0, 1=w74:i16)
        n64 = Boolean To (0,1)(Boolean=w68) -> (0, 1=w67:i16)
        n65 = Format Into String(format string="ScanType=%s\\nAverages=%u\\nRepetitions=%u\\nLensMode=%s\\nVoltageRange=%s\\nKineticEnergy=%f\\nPassEnergy=%f\\nCoilCurrent=%f\\nWorkFunction=%f\\nDetectorVoltage=%f\\nScreenVoltage=%f\\nConversionVoltage=%f\\nFocusDisplacement1=%f\\nFocusDisplacement2=%f\\nExposure=%u\\nGain=%u\\nBinning=%u\\nROIbottom=%u\\nROItop=%u\\nROIright=%u\\nROIleft=%u\\nDarkImg=%u\\nStartTime=%<%Y.%m.%d %H:%M:%S>T\\n\n", initial string=w65, "single" ("input 1"), w89, w88, w87, w86, w85, w84, w83, w82, w81, w80, w79, w78, w77, w76, w74, w73, w72, w71, w70, w69, w67, w66) -> ()  [unwired: 1 in, 2 out]
      }
      frame "scan" {
        n66 = Dequeue Element(queue=w154) -> ()  [unwired: 2 in, 4 out]
        n67 = local read "RunNumber"() -> (w162:u16)
        n68 = local read "BasePath"() -> (w163:path)
        n69 = local read "ROI Bottom"() -> (w140:i32)
        n70 = property on="ana_mode" class="Enum (strict)"() -> ("RingText.Text"=w149:string)  [unwired: 2 in, 2 out]
        n71 = property on="ana_voltrange" class="Enum (strict)"() -> ("RingText.Text"=w148:string)  [unwired: 2 in, 2 out]
        n72 = local read "cam_dark?"() -> (w146:bool)
        n73 = local read "phoib_I_1"() -> (w118:dbl)
        n74 = local read "phoib_I_2"() -> (w117:dbl)
        n75 = local read "phoib_I_3"() -> (w116:dbl)
        n76 = local read "phoib_I_4"() -> (w115:dbl)
        n77 = local read "phoib_I_5"() -> (w114:dbl)
        n78 = local read "phoib_I_6"() -> (w113:dbl)
        n79 = local read "phoib_I_7"() -> (w112:dbl)
        n80 = local read "phoib_I_8"() -> (w111:dbl)
        n81 = local read "phoib_I_9"() -> (w110:dbl)
        n82 = local read "cam_avgs"() -> (w151:i32)
        n83 = case shown="\"manip\"" "scan_selector" {
          tunnel: ["delay" ("input 1") "manipulator" ("input 1") "mirror" ("input 1") "voltage" ("input 1")] -> w144
          frame "delay", Default {
          }
          frame "manip" {
          }
          frame "mirror" {
          }
          frame "volt" {
          }
        }
        n84 = local read "meas_iter"() -> (w150:i32)
        n85 = local read "ROI Right"() -> (w138:i32)
        n86 = local read "cam_exp"() -> (w143:u32)
        n87 = local read "ROI Top"() -> (w139:i32)
        n88 = local read "ESP_t0"() -> (w109:dbl)
        n89 = local read "ROI Left"() -> (w137:i32)
        n90 = local read "binning"() -> (w141:u16)
        n91 = local read "gain"() -> (w147:bool)
        n92 = Increment(x=w162) -> (x+1=w164:u16)
        n93 = Current VI's Path() -> (path=w161:path)
        n94 = call "saverunnumber.vi"("RunNumber"=w164, "VI path"=w161) -> ()  [unwired: 10 in]
        n95 = local write "RunNumber"(w164) -> ()
        n96 = Boolean To (0,1)(Boolean=w147) -> (0, 1=w142:i16)
        n97 = Boolean To (0,1)(Boolean=w146) -> (0, 1=w136:i16)
        n98 = call "create_opti_path.vi"("RunNumber"=w164, "base path"=w163) -> ("Path"=w125:path)  [unwired: 2 in]
        n99 = call "create scan vectr.vi"("Table Control"="waypoints") -> ("Array"=w119:dbl[])
        n100 = Build Path(base path=w125, name or relative path="scanvector.txt") -> (appended path=w108:path)
        n101 = Build Path(base path=w125, name or relative path="info.txt") -> (appended path=w145:path)
        n102 = Format Into String(format string="ScanType:%s\\nAverages:%u\\nRepetitions:%u\\nLensMode:%s\\nVoltageRange:%s\\nExposure:%u\\nGain:%u\\nBinning:%u\\nROIbottom:%u\\nROItop:%u\\nROIright:%u\\nROIleft:%u\\nDarkImg:%u\\nKineticEnergy:%f\\nPassEnergy:%f\\nCoilCurrent:%f\\nWorkFunction:%f\\nDetectorVoltage:%f\\nScreenVoltage:%f\\nConversionVoltage:%f\\nFocusDisplacement1:%f\\nFocusDisplacement2:%f\\nTimeZero:%f", initial string=w145, w144, w151, w150, w149, w148, w143, w142, w141, w140, w139, w138, w137, w136, w118, w117, w116, w115, w114, w113, w112, w111, w110, w109) -> ()  [unwired: 1 in, 2 out]
        n103 = Unbundle(w134) -> ("queue out"=w126:refnum<queue>, "queue out"=w133:refnum<queue>, "queue out"=w132:refnum<queue>, "queue out"=w131:refnum<queue>, "queue out"=w130:refnum<queue>)
        n104 = for {
          tunnel: w119 -> [w307] mode=indexing
          tunnel: [w306] -> w127 mode=indexing
          tunnel: [w305] -> w128
          tunnel: w133 -> [w304]
          tunnel: w132 -> [w303]
          tunnel: w131 -> [w302]
          tunnel: w130 -> [w301]
          tunnel: "scan_selector" -> [w300]
          tunnel: w108 -> [w299]
          n105 = case shown="\"manip\"" w300 {
            tunnel: w307 -> [w315 w342 w355 w365]
            tunnel: [w313 w330 w352 w369] -> w305
            tunnel: [w319 w331 w353 w370] -> w306
            tunnel: w304 -> [w313 _ _ _]
            tunnel: w303 -> [_ w330 _ _]
            tunnel: w302 -> [_ _ _ w369]
            tunnel: w301 -> [_ _ w352 _]
            tunnel: w299 -> [w308 w325 w349 w366]
            frame "delay", Default {
              w321 = ":" ("string")
              n106 = local read "ESP_t0"() -> (w314:dbl)
              n107 = call "time2mm.vi"("fs[1]/ps[0]"=TRUE, "Offset (mm)"=w314, "time"=w315) -> ("position (mm)"=w310:dbl)
              n108 = local read "ESP Axis"() -> (w318:i32)
              n109 = Build Array(w310) -> (w309:dbl[])
              n110 = Number To Decimal String(number=w318) -> (decimal integer string=w317:string)  [unwired: 1 in]
              n111 = Number To Fractional String(number=w310) -> (F-format string=w323:string)  [unwired: 3 in]
              n112 = call-poly <vilib>:"Write Delimited Spreadsheet.vi"("file path (dialog if empty)"=w308, "format (%.3f)"="%.6f", "1D data"=w309, "append to file? (F)"=TRUE) -> ()  [unwired: 10 in, 2 out]
              n113 = Concatenate Strings("abs:" ("string"), w317, w321, w323, w321, "confirm" ("string")) -> (w319:string)
            }
            frame "manip" {
              n114 = call-poly <vilib>:"Vector Norm.vi"("Input Vector"="scan_manip_deltas") -> ("norm"=w344:dbl)  [unwired: 9 in, 1 out]
              n115 = Divide(x="scan_manip_deltas", y=w344) -> (x/y=w343:dbl[])
              n116 = Multiply(x=w343, y=w342) -> (x*y=w328:dbl[])
              n117 = Add(x="scan_manip_start", y=w328) -> (x+y=w324:dbl[])
              n118 = call-poly <vilib>:"Write Delimited Spreadsheet.vi"("file path (dialog if empty)"=w325, "format (%.3f)"="%.6f", "1D data"=w324, "append to file? (F)"=TRUE) -> ()  [unwired: 10 in, 2 out]
              n119 = Index Array(array=w324) -> (element #1=w333:dbl, element #2=w334:dbl, element #3=w335:dbl, element #4=w336:dbl, element #5=w337:dbl, element #6=w338:dbl)  [unwired: 6 in]
              n120 = Format Into String(format string="%g_%g_%g_%g_%g_%g", w333, w334, w335, w336, w337, w338) -> (resulting string=w340:string)  [unwired: 2 in, 1 out]
              n121 = Concatenate Strings("abs:" ("string"), w340, ":confirm" ("string")) -> (w331:string)
            }
            frame "mirror" {
              n122 = call-poly <vilib>:"Vector Norm.vi"("Input Vector"="scan_mirr_deltas") -> ("norm"=w363:dbl)  [unwired: 9 in, 1 out]
              n123 = Divide(x="scan_mirr_deltas", y=w363) -> (x/y=w362:dbl[])
              n124 = Multiply(x=w362, y=w355) -> (x*y=w351:dbl[])
              n125 = Add(x="scan_mirr_start", y=w351) -> (x+y=w348:dbl[])
              n126 = call-poly <vilib>:"Write Delimited Spreadsheet.vi"("file path (dialog if empty)"=w349, "format (%.3f)"="%.6f", "1D data"=w348, "append to file? (F)"=TRUE) -> ()  [unwired: 10 in, 2 out]
              n127 = Index Array(array=w348) -> (element #1=w358:dbl, element #2=w359:dbl)  [unwired: 2 in]
              n128 = Format Into String(format string="%g_%g", w358, w359) -> (resulting string=w361:string)  [unwired: 2 in, 1 out]
              n129 = Concatenate Strings("abs:" ("string"), w361, ":confirm" ("string")) -> (w353:string)
            }
            frame "volt" {
              n130 = local read "scan_volt_parameter"() -> (w373:string)
              n131 = Build Array(w365) -> (w364:dbl[])
              n132 = Number To Fractional String(number=w365) -> (F-format string=w371:string)  [unwired: 3 in]
              n133 = Concatenate Strings("setsgl:" ("string"), w373, ":" ("string"), w371) -> (w370:string)
              n134 = call-poly <vilib>:"Write Delimited Spreadsheet.vi"("file path (dialog if empty)"=w366, "format (%.3f)"="%.6f", "1D data"=w364, "append to file? (F)"=TRUE) -> ()  [unwired: 10 in, 2 out]
            }
          }
        }
        n135 = Build Path(base path=w125, name or relative path="RAW\\LUT.txt") -> (appended path=w123:path)
        n136 = call-poly <vilib>:"Write Delimited Spreadsheet.vi"("file path (dialog if empty)"=w123, "1D data"=string[] ["filename", "time", "delaystage", "delay", "X", "Y", "Z", "polar", "tilt", "azimuth", "mirrorX", "mirrorY", "KineticEnergy", "PassEnergy", "CoilCurrent", "WorkFunction", "DetectorVoltage", "ScreenVoltage", "ConversionVoltage", "FD1", "FD2"]) -> ("new file path (Not A Path if cancelled)"=w122:path)  [unwired: 12 in, 1 out]
        n137 = Get Date/Time In Seconds() -> (seconds since 1Jan1904=w135:timestamp)
        n138 = while {
          tunnel: w125 -> [w183]
          tunnel: w158 -> [w182]
          shift-right: [w181] -> w156
          shift-left: dbl[][][] [] -> [w180]
          tunnel: w155 -> [w179]
          tunnel: w135 -> [w178]
          tunnel: w128 -> [w177]
          tunnel: w127 -> [w176]
          tunnel: w126 -> [w175]
          shift-right: [w173] -> _
          shift-left: w122 -> [w174]
          shift-right: [w172] -> w120
          shift-left: w119 -> [w171]
          i -> [w170]
          stop <- w167 stop-if-true
          n139 = local read "meas_iter"() -> (w169:i32)
          n140 = for {
            N -> [w213]
            tunnel: w183 -> [w210]
            tunnel: w182 -> [w234]
            tunnel: w170 -> [w208]
            shift-right: [w223] -> w181
            shift-left: w180 -> [w230]
            tunnel: w179 -> [w225]
            tunnel: w178 -> [w212]
            tunnel: w177 -> [w204]
            tunnel: w176 -> [w203] mode=indexing
            tunnel: w175 -> [w202]
            shift-right: [w198] -> w173
            shift-left: w174 -> [w199]
            shift-right: [w194] -> w172
            shift-left: w171 -> [w194]
            tunnel: [w191] -> w166
            tunnel: w169 -> [w190]
            i -> [w209]
            stop <- "stop after step" stop-if-true
            n141 = Cancel Notification(0:w225) -> (11:w226:errorcluster)  [unwired: 1 in, 2 out]
            n142 = Enqueue Element(queue=w204, element=w203, error in (no error)=w226) -> (error out=w229:errorcluster)  [unwired: 1 in, 2 out]
            n143 = Equal To 0?(x=w209) -> (x = 0?=w233:bool)
            n144 = Equal To 0?(x=w208) -> (x = 0?=w232:bool)
            n145 = Get Date/Time In Seconds() -> (seconds since 1Jan1904=w200:timestamp)
            n146 = Wait on Notification(notifier=w225, error in (no error)=w229) -> (error out=w228:errorcluster)  [unwired: 2 in, 3 out]
            n147 = And(x=w233, y=w232) -> (x .and. y?=w231:bool)
            n148 = Enqueue Element(queue=w202, element="snap", error in (no error)=w228) -> (error out=w227:errorcluster)  [unwired: 1 in, 2 out]
            n149 = call "createFileStruc.vi"("i_iter"=w208, "i_delay"=w209, "meas_path"=w210) -> ("AVG file"=w205:path, "RAW file"=w196:path)  [unwired: 7 in]
            n150 = Dequeue Element(queue=w234, error in (no error)=w227) -> (element=w207:dbl[][], error out=w197:errorcluster)  [unwired: 1 in, 2 out]
            n151 = Strip Path(path=w196) -> (name=w195:string)  [unwired: 1 out]
            n152 = Array Size(array=w207) -> (size(s)=w238:i32[])
            n153 = call-poly <vilib>:"Write Delimited Spreadsheet.vi"("file path (dialog if empty)"=w196, "2D data"=w207, "error in (no error)"=w197) -> ()  [unwired: 11 in, 2 out]
            n154 = Index Array(array=w238) -> (element #1=w236:i32, element #2=w235:i32)  [unwired: 2 in]
            n155 = Subtract(x=w200, y=w212) -> (x-y=w216:dbl)
            n156 = flat-sequence {
              tunnel: "%s\\t%<%Y.%m.%d %H:%M:%S>T\\t%f\\t%f\\t%f\\t%f\\t%f\\t%f\\t%f\\t%f\\t%f\\t%f\\t%f\\t%f\\t%f\\t%f\\t%f\\t%f\\t%f\\t%f\\t%f" -> [w268]
              tunnel: w200 -> [w267]
              tunnel: w199 -> [w244]
              tunnel: [w243] -> w198
              tunnel: w197 -> [w240]
              tunnel: w195 -> [w239]
              frame #0 {
                n157 = local read "pos"() -> (w269:dbl[])
                n158 = local read "mirr_posX"() -> (w256:i32)
                n159 = local read "mirr_posY"() -> (w257:i32)
                n160 = local read "ESP_delay"() -> (w249:dbl)
                n161 = local read "phoib_I_1"() -> (w258:dbl)
                n162 = local read "phoib_I_2"() -> (w259:dbl)
                n163 = local read "phoib_I_3"() -> (w260:dbl)
                n164 = local read "phoib_I_4"() -> (w261:dbl)
                n165 = local read "phoib_I_5"() -> (w262:dbl)
                n166 = local read "phoib_I_6"() -> (w263:dbl)
                n167 = local read "phoib_I_7"() -> (w264:dbl)
                n168 = local read "phoib_I_8"() -> (w265:dbl)
                n169 = local read "phoib_I_9"() -> (w266:dbl)
                n170 = local read "ESP_pos"() -> (w248:dbl)
                n171 = Index Array(array=w269) -> (element #1=w250:dbl, element #2=w251:dbl, element #3=w252:dbl, element #4=w253:dbl, element #5=w254:dbl, element #6=w255:dbl)  [unwired: 6 in]
                n172 = Format Into String(format string=w268, error in=w240, w239, w267, w248, w249, w250, w251, w252, w253, w254, w255, w256, w257, w258, w259, w260, w261, w262, w263, w264, w265, w266) -> (resulting string=w246:string)  [unwired: 1 in, 1 out]
                n173 = Spreadsheet String To Array(format string="%s", spreadsheet string=w246, array type (2D Dbl)=string[] []) -> (array=w242:string[])  [unwired: 1 in]
                n174 = call-poly <vilib>:"Write Delimited Spreadsheet.vi"("file path (dialog if empty)"=w244, "1D data"=w242, "append to file? (F)"=TRUE) -> ("new file path (Not A Path if cancelled)"=w243:path)  [unwired: 11 in, 1 out]
              }
            }
            n175 = case shown="True" w231 {
              tunnel: w213 -> [_ w275]
              tunnel: [w270 w273] -> w237
              tunnel: w230 -> [w270 _]
              tunnel: w236 -> [_ w272]
              tunnel: w235 -> [_ w271]
              frame False {
              }
              frame True {
                n176 = Initialize Array(0.0 ("element"), w275, w272, w271) -> (w273:dbl[][][])
              }
            }
            n177 = Increment(x=w209) -> (x+1=w220:i32)
            "current scan" <- w220
            n178 = Increment(x=w208) -> (x+1=w219:i32)
            "current iteration" <- w219
            n179 = for {
              N: w236 -> [_]
              tunnel: w209 -> [w282]
              shift-right: [w280] -> w223
              shift-left: w237 -> [w283]
              tunnel: w208 -> [w278]
              shift-right: [w277] -> w206
              shift-left: w207 -> [w279]
              tunnel: w235 -> [w276]
              i -> [w281]
              n180 = for {
                N: w276 -> [_]
                tunnel: w282 -> [w290]
                tunnel: w281 -> [w287]
                shift-right: [w289] -> w280
                shift-left: w283 -> [w291]
                tunnel: w278 -> [w285]
                shift-right: [w284] -> w277
                shift-left: w279 -> [w288]
                i -> [w286]
                n181 = in-place {
                  in-place-border: w285 -> [w297]
                  n182 = in-place-array #1(w291, w290, w287, w286) -> (w298:dbl)
                  n183 = in-place-array #2(w288, w287, w286) -> (w295:dbl)
                  n184 = Multiply(x=w298, y=w297) -> (x*y=w296:dbl)
                  n185 = Increment(x=w297) -> (x+1=w293:i32)
                  n186 = Add(x=w296, y=w295) -> (x+y=w294:dbl)
                  n187 = Divide(x=w294, y=w293) -> (x/y=w292:dbl)
                  n188 = in-place-array #1(w292) -> (w289:dbl[][][])  [unwired: 3 out]
                  n189 = in-place-array #2(w292) -> (w284:dbl[][])  [unwired: 2 out]
                }
              }
            }
            n190 = Multiply(x=w213, y=w208) -> (x*y=w215:i32)
            n191 = Multiply(x=w213, y=w190) -> (x*y=w211:i32)
            n192 = Divide(x=w220, y=w213) -> (x/y=→"scan":dbl)
            n193 = Divide(x=w219, y=w190) -> (x/y=→"iteration":dbl)
            n194 = Add(x=w209, y=w215) -> (x+y=w214:i32)
            n195 = Divide(x=w216, y=w214) -> (x/y=w186:dbl)
            n196 = Multiply(x=w186, y=w211) -> (x*y=w189:dbl)
            n197 = local write "time/step [s]"(w186) -> ()
            n198 = local write "duration [HH:MM:SS]"(w189) -> ()
            n199 = property on="mainimg" class="IntGraph (strict)"() -> ("CrsrLis"=w222:T5)  [unwired: 2 in, 2 out]
            n200 = call-poly <vilib>:"Write Delimited Spreadsheet.vi"("file path (dialog if empty)"=w205, "2D data"=w206) -> ()  [unwired: 12 in, 2 out]
            n201 = call "processData.vi"("Cursor List"=w222, "data in"=w223) -> ("Angle Chart"=→"anglegraph":dbl[][], "Energy Chart"=→"energygraph":dbl[][], "Intensity Chart"=w221:dbl[])  [unwired: 1 in]
            n202 = Bundle("Array"=w194, "Intensity Chart"=w221) -> (w185:cluster{"Array":dbl[], "Intensity Chart":dbl[]})  [unwired: 1 in]
            n203 = Build Array(w185) -> (→"intensitygraph":T2)
            n204 = Or(x="stop after iteration", y="stop after step") -> (x .or. y?=w191:bool)
          }
          n205 = Increment(x=w170) -> (x+1=w168:i32)
          n206 = Greater Or Equal?(x=w168, y=w169) -> (x >= y?=w165:bool)
          n207 = Or(x=w166, y=w165) -> (x .or. y?=w167:bool)
        }
      }
      frame "refresh" {
        n208 = Dequeue Element(queue=w381) -> ()  [unwired: 2 in, 4 out]
        n209 = property on="mainimg" class="IntGraph (strict)"() -> ("CrsrLis"=w387:T5)  [unwired: 2 in, 2 out]
        n210 = call "processData.vi"("Cursor List"=w387, "data in"=w386) -> ("Angle Chart"=w384:dbl[][], "Energy Chart"=w385:dbl[][], "Intensity Chart"=w382:dbl[])  [unwired: 1 in]
        n211 = Bundle("Array"=w383, "Intensity Chart"=w382) -> (w380:cluster{"Array":dbl[], "Intensity Chart":dbl[]})  [unwired: 1 in]
        n212 = Build Array(w380) -> (w379:T2)
        n213 = local write "energygraph"(w385) -> ()
        n214 = local write "intensitygraph"(w379) -> ()
        n215 = local write "anglegraph"(w384) -> ()
      }
    }
  }
  n216 = while {
    tunnel: w14 -> [w395]
    tunnel: w13 -> [w394]
    tunnel: w12 -> [w393]
    tunnel: w11 -> [w392]
    tunnel: w16 -> [w390]
    tunnel: w23 -> [w391]
    tunnel: w3 -> [w389]
    tunnel: w4 -> [w388]
    stop <- w396 stop-if-true
    n217 = event shown="[13] \"gauss fit\": Value Change" {
      selector: _ -> [_ _ _ _ _ _ _ _ _ _ _ _ _ _ _ _ _ _ _ _ _ _ _ _ _ _ _ _ _ _]
      dyn-events: _ -> [_ _ _ _ _ _ _ _ _ _ _ _ _ _ _ _ _ _ _ _ _ _ _ _ _ _ _ _ _ _]
      timeout: _ -> [_ _ _ _ _ _ _ _ _ _ _ _ _ _ _ _ _ _ _ _ _ _ _ _ _ _ _ _ _ _]
      tunnel: [_ TRUE _ _ _ _ _ _ _ _ _ _ _ _ _ _ _ _ _ _ _ _ _ _ _ _ _ _ _ _] -> w396
      tunnel: w395 -> [_ w408 w421 _ _ _ _ _ w447 w449 _ _ _ _ _ _ _ _ _ _ _ _ _ _ _ _ _ _ _ _]
      tunnel: w394 -> [_ w407 _ w425 _ _ _ _ _ _ _ _ _ _ _ _ _ _ _ _ w524 _ _ w546 _ _ _ _ _ _]
      tunnel: w393 -> [_ w406 _ _ w431 _ _ _ _ _ _ _ _ _ _ _ _ w499 w514 w516 _ _ _ _ _ _ _ _ _ _]
      tunnel: w392 -> [_ w405 _ _ _ w437 w443 w444 _ _ _ _ _ _ _ _ _ _ _ _ _ _ _ _ _ _ _ _ _ _]
      tunnel: w391 -> [_ w414 _ _ _ _ _ _ _ _ _ _ _ _ _ _ _ _ _ _ _ _ _ _ _ _ _ _ _ _]
      tunnel: w390 -> [_ w404 _ _ _ _ _ _ _ _ w451 w453 _ _ _ _ _ _ _ _ _ _ _ _ _ _ _ w565 _ _]
      tunnel: w389 -> [_ w413 _ _ _ _ _ _ _ _ _ _ _ _ _ _ _ _ _ _ _ _ _ _ _ _ _ _ _ _]
      tunnel: w388 -> [_ w403 _ _ _ _ _ _ _ _ _ _ _ _ w477 _ _ _ _ _ _ _ _ _ _ _ _ _ w567 w588]
      event Timeout {
        n218 = event-data() -> ()  [unwired: 1 in, 1 out]
      }
      event "main_close": Value Change {
        w409 = "close" ("element")
        w410 = "release" ("element")
        n219 = event-data() -> ()  [unwired: 1 in, 1 out]
        n220 = Flush Queue(queue=w408) -> (queue out=w402:refnum<queue>)  [unwired: 1 in, 2 out]
        n221 = Flush Queue(queue=w407) -> (queue out=w401:refnum<queue>)  [unwired: 1 in, 2 out]
        n222 = Flush Queue(queue=w406) -> (queue out=w400:refnum<queue>)  [unwired: 1 in, 2 out]
        n223 = Flush Queue(queue=w405) -> (queue out=w399:refnum<queue>)  [unwired: 1 in, 2 out]
        n224 = Flush Queue(queue=w404) -> (queue out=w398:refnum<queue>)  [unwired: 1 in, 2 out]
        n225 = Flush Queue(queue=w403) -> (queue out=w397:refnum<queue>)  [unwired: 1 in, 2 out]
        n226 = Release Notifier(notifier=w413) -> ()  [unwired: 2 in, 3 out]
        n227 = Release Queue(queue=w414) -> ()  [unwired: 2 in, 3 out]
        n228 = Enqueue Element(queue=w402, element=w410) -> (queue out=w418:refnum<queue>)  [unwired: 2 in, 2 out]
        n229 = Enqueue Element(queue=w401, element=w410) -> (queue out=w417:refnum<queue>)  [unwired: 2 in, 2 out]
        n230 = Enqueue Element(queue=w400, element=w410) -> (queue out=w416:refnum<queue>)  [unwired: 2 in, 2 out]
        n231 = Enqueue Element(queue=w399, element=w410) -> (queue out=w415:refnum<queue>)  [unwired: 2 in, 2 out]
        n232 = Enqueue Element(queue=w397, element=w410) -> (queue out=w412:refnum<queue>, error out=w411:errorcluster)  [unwired: 2 in, 1 out]
        n233 = Enqueue Element(queue=w418, element=w409) -> ()  [unwired: 2 in, 3 out]
        n234 = Enqueue Element(queue=w417, element=w409) -> ()  [unwired: 2 in, 3 out]
        n235 = Enqueue Element(queue=w416, element=w409) -> ()  [unwired: 2 in, 3 out]
        n236 = Enqueue Element(queue=w415, element=w409) -> ()  [unwired: 2 in, 3 out]
        n237 = Enqueue Element(queue=w398, element=w409) -> ()  [unwired: 2 in, 3 out]
        n238 = Enqueue Element(queue=w412, element=w409, error in (no error)=w411) -> ()  [unwired: 1 in, 3 out]
      }
      event "cam_release", "cam_init": Value Change {
        n239 = event-data() -> ()  [unwired: 1 in, 2 out]
        n240 = Select(t="init" ("name (unnamed)"), s="cam_init", f="release" ("name (unnamed)")) -> (s? t:f=w420:string)
        n241 = Enqueue Element(queue=w421, element=w420) -> ()  [unwired: 2 in, 3 out]
      }
      event "ESP_release", "ESP_init": Value Change {
        n242 = event-data() -> ()  [unwired: 1 in, 2 out]
        n243 = Select(t="init" ("name (unnamed)"), s="ESP_init", f="release" ("name (unnamed)")) -> (s? t:f=w429:string)
        n244 = Enqueue Element(queue=w425, element=w429) -> ()  [unwired: 2 in, 3 out]
      }
      event "manip_init", "manip_release": Value Change {
        n245 = event-data() -> ()  [unwired: 1 in, 2 out]
        n246 = Flush Queue(queue=w431) -> (queue out=w430:refnum<queue>)  [unwired: 1 in, 2 out]
        n247 = Select(t="init" ("name (unnamed)"), s="manip_init", f="release" ("name (unnamed)")) -> (s? t:f=w433:string)
        n248 = Enqueue Element(queue=w430, element=w433) -> ()  [unwired: 2 in, 3 out]
      }
      event "phoib_release", "phoib_init": Value Change {
        n249 = event-data() -> ()  [unwired: 1 in, 2 out]
        n250 = Flush Queue(queue=w437) -> (queue out=w436:refnum<queue>)  [unwired: 1 in, 2 out]
        n251 = Select(t="init" ("name (unnamed)"), s="phoib_init", f="release" ("name (unnamed)")) -> (s? t:f=w439:string)
        n252 = Enqueue Element(queue=w436, element=w439) -> ()  [unwired: 2 in, 3 out]
      }
      event "phoib_standby": Value Change {
        n253 = event-data() -> ()  [unwired: 1 in, 2 out]
        n254 = Enqueue Element(queue=w443, element="standby") -> ()  [unwired: 2 in, 3 out]
      }
      event "phoib_set": Value Change {
        n255 = event-data() -> ()  [unwired: 1 in, 2 out]
        n256 = Enqueue Element(queue=w444, element="set") -> ()  [unwired: 2 in, 3 out]
      }
      event "cam_dark": Value Change {
        n257 = event-data() -> ()  [unwired: 1 in, 2 out]
        n258 = Enqueue Element(queue=w447, element="dark") -> ()  [unwired: 2 in, 3 out]
      }
      event "ROI Left", "ROI Right", "ROI Top", "ROI Bottom", "cam_exp", "binning", "gain": Value Change {
        n259 = event-data() -> ()  [unwired: 1 in, 1 out]
        n260 = Enqueue Element(queue=w449, element="set") -> ()  [unwired: 2 in, 3 out]
      }
      event "cam_saveimg": Value Change {
        n261 = event-data() -> ()  [unwired: 1 in, 1 out]
        n262 = Enqueue Element(queue=w451, element="single") -> ()  [unwired: 2 in, 3 out]
      }
      event "scan_go": Value Change {
        n263 = event-data() -> ()  [unwired: 1 in, 1 out]
        n264 = Enqueue Element(queue=w453, element="scan") -> ()  [unwired: 2 in, 3 out]
      }
      event "meas_iter", "waypoints": Value Change {
        n265 = event-data() -> ()  [unwired: 1 in, 6 out]
        n266 = local read "waypoints"() -> (w465:string[][])
        n267 = local read "meas_iter"() -> (w459:i32)
        n268 = local read "binning"() -> (w462:u16)
        n269 = call "create scan vectr.vi"("Table Control"=w465) -> ("Array"=w464:dbl[])
        n270 = Index Array(array=dbl[] [8.79, 2.2, 0.553, 0.138], index=w462) -> (element=w458:dbl)
        n271 = Array Size(array=w464) -> (size(s)=w461:i32)
        "measpoints" <- w461
        n272 = Multiply(x=w461, y=w459) -> (x*y=w456:i32)
        "total steps" <- w456
        n273 = Multiply(x=w456, y="time/step [s]") -> (x*y=→"duration [HH:MM:SS]":dbl)
        n274 = Multiply(x=w461, y=w458) -> (x*y=→"RAM [MB]":dbl)
        n275 = Multiply(x=w456, y=w458) -> (x*y=→"disk [MB]":dbl)
      }
      event "gauss fit": Value Change {
        w475 = T6 2 items=["Least Square", "Least Absolute Residual", "Bisquare"] ("method")
        n276 = event-data() -> ()  [unwired: 1 in, 6 out]
        n277 = local read "intensitygraph"() -> (w467:T2)
        n278 = Index Array(array=w467) -> (element=w466:cluster{"Array":dbl[], "Intensity Chart":dbl[]})  [unwired: 1 in]
        n279 = Unbundle(w466) -> ("Array"=w472:dbl[], "Intensity Chart"=w473:dbl[])
        n280 = call <vilib>:"Gaussian Peak Fit.vi"("Y"=w473, "X"=w472, "method"=w475) -> ("Best Gaussian Fit"=w471:dbl[], "center"=→"center":dbl)  [unwired: 6 in, 5 out]
        n281 = Bundle("Array"=w472, "Intensity Chart"=w473) -> (w470:cluster{"Array":dbl[], "Intensity Chart":dbl[]})  [unwired: 1 in]
        n282 = Bundle("Array"=w472, "Best Gaussian Fit"=w471) -> (w469:T7)  [unwired: 1 in]
        n283 = Build Array(w470, w469) -> (w468:T8)
        n284 = local write "intensitygraph"(w468) -> ()
      }
      event "mirr_go": Value Change {
        n285 = event-data() -> ()  [unwired: 1 in, 1 out]
        n286 = Index Array(array="mirr_dest") -> (element #1=w482:i32, element #2=w481:i32)  [unwired: 2 in]
        n287 = Format Into String(format string="%g_%g", w482, w481) -> (resulting string=w479:string)  [unwired: 2 in, 1 out]
        n288 = Concatenate Strings("abs:" ("string"), w479) -> (w476:string)
        n289 = Enqueue Element(queue=w477, element=w476) -> ()  [unwired: 2 in, 3 out]
      }
      event "scan_manip_setstart": Value Change {
        n290 = event-data() -> ()  [unwired: 1 in, 1 out]
        n291 = local read "pos"() -> (w484:dbl[])
        n292 = local write "scan_manip_start"(w484) -> ()
      }
      event "scan_mirr_setstart": Value Change {
        n293 = event-data() -> ()  [unwired: 1 in, 1 out]
        n294 = local read "mirr_posX"() -> (w487:i32)
        n295 = local read "mirr_posY"() -> (w486:i32)
        n296 = Build Array(w487, w486) -> (w485:i32[])
        n297 = local write "scan_mirr_start"(w485) -> ()
      }
      event "Move Abs": Value Change {
        n298 = event-data() -> ()  [unwired: 1 in, 1 out]
        n299 = Index Array(array="dest") -> (element #1=w497:dbl, element #2=w496:dbl, element #3=w495:dbl, element #4=w494:dbl, element #5=w493:dbl, element #6=w492:dbl)  [unwired: 6 in]
        n300 = Format Into String(format string="%g_%g_%g_%g_%g_%g", w497, w496, w495, w494, w493, w492) -> (resulting string=w490:string)  [unwired: 2 in, 1 out]
        n301 = Concatenate Strings("abs:" ("string"), w490) -> (w489:string)
        n302 = Enqueue Element(queue=w499, element=w489) -> ()  [unwired: 2 in, 3 out]
      }
      event "ManipRel +", "ManipRel -": Value Change {
        n303 = event-data() -> ()  [unwired: 1 in, 2 out]
        n304 = Negate(x="manip_deltas") -> (-x=w502:dbl[])
        n305 = Select(t="manip_deltas", s="ManipRel +", f=w502) -> (s? t:f=w500:dbl[])
        n306 = Index Array(array=w500) -> (element #1=w506:dbl, element #2=w507:dbl, element #3=w508:dbl, element #4=w509:dbl, element #5=w510:dbl, element #6=w511:dbl)  [unwired: 6 in]
        n307 = Format Into String(format string="%g_%g_%g_%g_%g_%g", w506, w507, w508, w509, w510, w511) -> (resulting string=w513:string)  [unwired: 2 in, 1 out]
        n308 = Concatenate Strings("rel:" ("string"), w513) -> (w504:string)
        n309 = Enqueue Element(queue=w514, element=w504) -> ()  [unwired: 2 in, 3 out]
      }
      event "stop manip": Value Change {
        n310 = event-data() -> ()  [unwired: 1 in, 1 out]
        n311 = Enqueue Element(queue=w516, element="stop") -> ()  [unwired: 2 in, 3 out]
      }
      event "ESP_go": Value Change {
        w518 = ":" ("string")
        n312 = event-data() -> ()  [unwired: 1 in, 1 out]
        n313 = local read "ESP Axis"() -> (w517:i32)
        n314 = Number To Decimal String(number=w517) -> (decimal integer string=w520:string)  [unwired: 1 in]
        n315 = Number To Fractional String(number="ESP_dest") -> (F-format string=w519:string)  [unwired: 3 in]
        n316 = Concatenate Strings("abs:" ("string"), w520, w518, w519, w518) -> (w523:string)
        n317 = Enqueue Element(queue=w524, element=w523) -> ()  [unwired: 2 in, 3 out]
      }
      event "ESP_set_t0": Value Change {
        n318 = event-data() -> ()  [unwired: 1 in, 1 out]
        n319 = Current VI's Path() -> (path=w535:path)
        n320 = Strip Path(path=w535) -> (stripped path=w533:path)  [unwired: 1 out]
        n321 = Strip Path(path=w533) -> (stripped path=w532:path)  [unwired: 1 out]
        n322 = local read "ESP_pos"() -> (w534:dbl)
        "ESP_t0" <- w534
        n323 = Number To Fractional String(number=w534) -> (F-format string=w527:string)  [unwired: 3 in]
        n324 = Build Path(base path=w532, name or relative path="t0.txt") -> (appended path=w529:path)
        n325 = Get Date/Time In Seconds() -> (seconds since 1Jan1904=w531:timestamp)
        n326 = Format Date/Time String(time format string (%c)="%Y.%m.%d %H:%M", seconds (now)=w531) -> (date/time string=w528:string)  [unwired: 1 in]
        n327 = Build Array(w528, w527) -> (w526:string[])
        n328 = call-poly <vilib>:"Write Delimited Spreadsheet.vi"("file path (dialog if empty)"=w529, "1D data"=w526, "append to file? (F)"=TRUE) -> ()  [unwired: 11 in, 2 out]
      }
      event "ESP_opent0file": Value Change {
        n329 = event-data() -> ()  [unwired: 1 in, 6 out]
        n330 = Current VI's Path() -> (path=w539:path)
        n331 = Strip Path(path=w539) -> (stripped path=w538:path)  [unwired: 1 out]
        n332 = Strip Path(path=w538) -> (stripped path=w540:path)  [unwired: 1 out]
        n333 = call <vilib>:"System Exec.vi"("wait until completion? (T)"=FALSE, "working directory"=w540, "command line"="notepad t0.txt") -> ()  [unwired: 5 in, 4 out]
      }
      event "ESP_+", "ESP_-": Value Change {
        n334 = event-data() -> ()  [unwired: 1 in, 6 out]
        n335 = local read "ESP Axis"() -> (w542:i32)
        n336 = Negate(x="ESP_delta") -> (-x=w549:dbl)
        n337 = Select(t="ESP_delta", s="ESP_+", f=w549) -> (s? t:f=w547:dbl)
        n338 = Number To Decimal String(number=w542) -> (decimal integer string=w545:string)  [unwired: 1 in]
        n339 = Number To Fractional String(number=w547) -> (F-format string=w543:string)  [unwired: 3 in]
        n340 = Concatenate Strings("rel:" ("string"), w545, ":" ("string"), w543) -> (w552:string)
        n341 = Enqueue Element(queue=w546, element=w552) -> ()  [unwired: 2 in, 3 out]
      }
      event "ESP_dest": Value Change {
        n342 = event-data() -> ()  [unwired: 1 in, 6 out]
        n343 = local read "ESP_dest"() -> (w556:dbl)
        n344 = local read "ESP_t0"() -> (w555:dbl)
        n345 = call "mm2time.vi"("fs?"=TRUE ("fs[1]/ps[0]"), "Offset (mm)"=w555, "distance (mm)"=w556) -> ("time in fs/ps seconds"=w553:dbl)
        n346 = local write "ESP_dest_t"(w553) -> ()
      }
      event "ESP_dest_t": Value Change {
        n347 = event-data() -> ()  [unwired: 1 in, 1 out]
        n348 = local read "ESP_t0"() -> (w559:dbl)
        n349 = call "time2mm.vi"("fs[1]/ps[0]"=TRUE, "Offset (mm)"=w559, "time"="ESP_dest_t") -> ("position (mm)"=w557:dbl)
        n350 = local write "ESP_dest"(w557) -> ()
      }
      event "load delay table": Value Change {
        n351 = event-data() -> ()  [unwired: 1 in, 6 out]
        n352 = call-poly <vilib>:"Read Delimited Spreadsheet.vi"() -> ("all rows"=w562:string[][], "error out"=w561:errorcluster)  [unwired: 10 in, 4 out]
        n353 = case shown="No Error" w561 {
          tunnel: w562 -> [w563 _]
          frame No Error {
            n354 = local write "waypoints"(w563) -> ()
          }
          frame Error {
          }
        }
      }
      event "mainimg": Cursor Release {
        n355 = event-data() -> ()  [unwired: 1 in, 1 out]
        n356 = Enqueue Element(queue=w565, element="refresh") -> ()  [unwired: 2 in, 3 out]
      }
      event "mirr_init", "mirr_release": Value Change {
        n357 = event-data() -> ()  [unwired: 1 in, 6 out]
        n358 = Flush Queue(queue=w567) -> (queue out=w568:refnum<queue>)  [unwired: 1 in, 2 out]
        n359 = Select(t="init" ("name (unnamed)"), s="mirr_init", f="release" ("name (unnamed)")) -> (s? t:f=w569:string)
        n360 = Enqueue Element(queue=w568, element=w569) -> ()  [unwired: 2 in, 3 out]
      }
      event "mirr_X-", "mirr_X+", "mirr_Y+", "mirr_Y-": Value Change {
        n361 = event-data() -> ()  [unwired: 1 in, 1 out]
        n362 = local read "mirr_X#"() -> (w579:u8)
        n363 = local read "mirr_Y#"() -> (w578:u8)
        n364 = Or(x="mirr_X+", y="mirr_X-") -> (x .or. y?=w580:bool)
        n365 = Or(x="mirr_X-", y="mirr_Y-") -> (x .or. y?=w586:bool)
        n366 = Negate(x="mirr_rel") -> (-x=w585:i32)
        n367 = Select(t=w579, s=w580, f=w578) -> (s? t:f=w577:u8)
        n368 = Select(t=w585, s=w586, f="mirr_rel") -> (s? t:f=w574:i32)
        n369 = Number To Decimal String(number=w577) -> (decimal integer string=w576:string)  [unwired: 1 in]
        n370 = Number To Decimal String(number=w574) -> (decimal integer string=w573:string)  [unwired: 1 in]
        n371 = Concatenate Strings("rel:" ("string"), w576, ":" ("string"), w573) -> (w572:string)
        n372 = Enqueue Element(queue=w588, element=w572) -> ()  [unwired: 2 in, 3 out]
      }
    }
  }
  n373 = while {
    tunnel: w14 -> [w615]
    shift-right: [w609] -> _
    shift-left: _ -> [w608]
    shift-right: [w607] -> _
    shift-left: _ -> [w605]
    shift-right: [w606] -> _
    shift-left: _ -> [w604]
    shift-right: [w601] -> _
    shift-left: 0 -> [w602]
    shift-right: [w600] -> _
    shift-left: _ -> [w599]
    shift-right: [w598] -> _
    shift-left: _ -> [w597]
    tunnel: w23 -> [w596]
    shift-right: [w595] -> _
    shift-left: _ -> [w594]
    shift-right: [w592] -> _
    shift-left: _ -> [w591]
    shift-right: [w590] -> _
    shift-left: _ -> [w589]
    i -> [w593]
    stop <- w603 stop-if-true
    # "cam"
    n374 = Preview Queue Element(queue=w615, timeout in ms (-1)=w602) -> (queue out=w614:refnum<queue>, element=w613:string)  [unwired: 1 in, 2 out]
    n375 = Match Pattern(string=w613, regular expression=":") -> (before substring=w610:string, after substring=w611:string)  [unwired: 1 in, 2 out]
    n376 = case shown="\"idle\", Default" w610 {
      tunnel: w614 -> [w627 w659 w692 w705 _ w793 w823 w888]
      tunnel: w611 -> [_ _ _ _ _ _ _ _]
      tunnel: [w621 w646 w691 w703 w746 w790 w808 w886] -> w609
      tunnel: w608 -> [_ _ w691 w703 w746 w790 w808 w886]
      tunnel: [w626 w660 u64 0 ("Hout") w702 w750 w791 w818 w885] -> w607
      tunnel: [w628 w661 w688 w701 w751 w792 w809 w884] -> w606
      tunnel: w605 -> [_ w663 w690 w702 w753 w795 w820 w885]
      tunnel: w604 -> [_ w662 _ w701 w752 w794 w819 w884]
      tunnel: [_ _ _ TRUE _ _ _ _] -> w603
      tunnel: [_ _ -1 _ _ _ _ -1] -> w601
      tunnel: [w620 w647 _ _ w760 _ _ _] -> w600
      tunnel: w599 -> [w620 w647 _ _ w759 _ _ _]
      tunnel: [w621 w649 w686 w700 w755 w784 w821 w883] -> w598
      tunnel: w597 -> [_ w649 w686 w700 w755 _ w821 w883]
      tunnel: w596 -> [_ _ _ _ _ _ w812 _]
      tunnel: [w618 w644 w685 w698 w713 w781 w815 w882] -> w595
      tunnel: w594 -> [w618 w644 w685 w698 w748 w781 w815 w882]
      tunnel: w593 -> [_ _ _ _ w721 _ _ _]
      tunnel: [w619 w645 w684 w699 w747 w780 w814 w881] -> w592
      tunnel: w591 -> [w619 w645 w684 w699 w720 w780 w814 w881]
      tunnel: [w617 w641 refnum<k21> refnum ("task out") w697 w706 w779 w805 w880] -> w590
      tunnel: w589 -> [_ w641 w683 w697 w706 w779 w806 w880]
      frame "init" {
        w621 = u16[][] []
        n377 = flat-sequence {
          tunnel: [w630] -> w625
          tunnel: [w631] -> w624
          tunnel: [w639] -> w626
          tunnel: [w640] -> w628
          tunnel: w625 -> [w640]
          tunnel: w624 -> [w639]
          frame #0 {
            n378 = local write "cam_con?"(FALSE ("cam_con?")) -> ()
          }
          frame #1 {
            n379 = call "SCInitBoard.vi"("boardnr"="board number") -> ("Hout"=w634:u32, "error out"=w635:errorcluster)  [unwired: 1 in, 1 out]
            n380 = call "SCSetupCamera.vi"("Handle"=w634, "error in (no error)"=w635) -> ("Hout"=w636:u64, "error out"=w637:errorcluster)  [unwired: 1 out]
            n381 = call "SCStopCOC.vi"("error in (no error)"=w637, "Stop mode"=0, "Handle"=w636) -> ("error out"=w630:errorcluster, "Hout"=w631:u64)
          }
          frame #2 {
            n382 = local write "cam_con?"(TRUE ("cam_con?")) -> ()
          }
        }
        n383 = Dequeue Element(queue=w627) -> (queue out=w623:refnum<queue>)  [unwired: 2 in, 3 out]
        n384 = Enqueue Element At Opposite End(queue=w623, element="set") -> ()  [unwired: 2 in, 3 out]
        n385 = call-poly <vilib>:"DAQmx Create Virtual Channel.vi"("lines"=tag "Dev2/port0/line7") -> ("task out"=w617:refnum<k21>)  [unwired: 13 in, 1 out]
      }
      frame "set" {
        n386 = Dequeue Element(queue=w659) -> ()  [unwired: 2 in, 4 out]
        n387 = call "SCStopCOC.vi"("error in (no error)"=w662, "Stop mode"=0, "Handle"=w663) -> ("error out"=w678:errorcluster, "Hout"=w677:u64)
        n388 = Bundle By Name(cluster=cluster{"Delay":dbl, "Exposure ":dbl} {"Delay"=0.0, "Exposure "=0.0} ("Delay and exposure"), "Exposure"="cam_exp") -> (w656:cluster{"Delay":dbl, "Exposure ":dbl})
        n389 = Bundle By Name(cluster=T9 {"Camera type"=0, "Operating mode\nHP & QE / HS & DiCam Pro "=0, "Frame trigger \n(High Performance and QE only)"=0, "Sequence trigger"=0, "Low Light\n(QE only)"=FALSE, "Gain"=FALSE, "Horzontal\nbinning"=0, "Vertical\nbinning "=0, "ROI Left"=1, "ROI Right"=20, "ROI Top"=1, "ROI Bottom"=15} ("Camera controls"), "Operating mode\nHP & QE / HS & DiCam Pro"="Operating mode\nHP & QE / HS & DiCam Pro", "Horzontal\nbinning"="binning", "Vertical\nbinning"="binning", "ROI Left"="ROI Left", "ROI Right"="ROI Right", "ROI Top"="ROI Top", "ROI Bottom"="ROI Bottom", "Gain"="gain", "Frame trigger \n(High Performance and QE only)"="Frame trigger \n(High Performance and QE only)") -> (w673:T9)
        n390 = call "New delay and exposure forma.vi"("Operating mode\nHP & QE / HS & DiCam Pro"="Operating mode\nHP & QE / HS & DiCam Pro", "Delay and exposure"=w656) -> ("Output table"=w674:string)  [unwired: 3 in]
        n391 = call "SCSetCoC.vi"("error in (no error)"=w678, "Delay and exposure table"=w674, "Camera controls"=w673, "Handle"=w677) -> ("error out"=w666:errorcluster, "Hout"=w665:u64)  [unwired: 1 out]
        n392 = call "SCGetImageSize.vi"("Handle"=w665, "error in (no error)"=w666) -> ("Hout"=w664:u64, "error out"=w648:errorcluster, "Horizontal size"=w653:i32, "Vertical size"=w652:i32)  [unwired: 2 out]
        n393 = Greater?(x=w653, y=w652) -> (0:w654:bool)
        n394 = Initialize Array(u16 0 ("dimension size"), w652, w653) -> (w646:u16[][])
        n395 = call "SCRun.vi"("error in (no error)"=w648, "Run mode"=0, "Handle"=w664) -> ("error out"=w661:errorcluster, "Hout"=w660:u64)  [unwired: 1 out]
        n396 = Select(t=w653, s=w654, f=w652) -> (s? t:f=w651:i32)
        n397 = property on="mainimg" class="IntGraph (strict)"("XScale.Maximum"=w651, "YScale.Maximum"=w651) -> ()  [unwired: 2 in, 2 out]
      }
      frame "release" {
        n398 = Dequeue Element(queue=w692) -> (queue out=w679:refnum<queue>)  [unwired: 2 in, 3 out]
        n399 = flat-sequence {
          tunnel: w690 -> [w694]
          tunnel: [w693] -> w687
          tunnel: [w696] -> w688
          tunnel: w687 -> [w696]
          frame #0 {
            n400 = call "SCCloseBoard.vi"("Handle"=w694) -> ("error out"=w693:errorcluster)  [unwired: 1 in, 2 out]
          }
          frame #1 {
            n401 = local write "cam_con?"(FALSE ("cam_con?")) -> ()
          }
        }
        n402 = Enqueue Element(queue=w679, element="suspend") -> ()  [unwired: 2 in, 3 out]
        n403 = call <vilib>:"DAQmx Clear Task.vi"("task in"=w683) -> ()  [unwired: 14 in, 1 out]
      }
      frame "close" {
        n404 = Release Queue(queue=w705) -> ()  [unwired: 2 in, 3 out]
      }
      frame "idle", Default {
        n405 = call "grabimg.vi"("array in"=w746, "error in"=w752, "Hin"=w753) -> ("error out"=w751:errorcluster, "imgdata"=w749:i32[][], "Hout"=w750:u64)  [unwired: 6 in]
        n406 = local read "lower threshold"() -> (w744:i32)
        n407 = case shown="False" "cam_dark?" {
          tunnel: w755 -> [_ w778]
          tunnel: [w775 w777] -> w745
          tunnel: w749 -> [w775 w776]
          frame False {
          }
          frame True {
            n408 = Subtract(x=w776, y=w778) -> (x-y=w777:dbl[][])
          }
        }
        n409 = call "filtr_b.vi"("threshold"=w744, "input array"=w745) -> ("output array"=w736:dbl[][])  [unwired: 9 in]
        n410 = call <vilib>:"High Resolution Relative Seconds.vi"() -> ("relative seconds"=w760:dbl)
        n411 = Subtract(x=w760, y=w759) -> (x-y=w758:dbl)
        n412 = Array Size(array=w736) -> (size(s)=w735:i32[])
        n413 = Reciprocal(x=w758) -> (1/x=→"cam_fps":dbl)
        n414 = Index Array(array=w735) -> (element #1=w730:i32, element #2=w729:i32)  [unwired: 2 in]
        n415 = Subtract(x=w721, y=w720) -> (x-y=w719:i32)
        n416 = Less Or Equal?(x="pics2avg", y=w719) -> (x <= y?=w742:bool)
        n417 = And(x="reset every n pics", y=w742) -> (x .and. y?=w740:bool)
        n418 = Not(x=w740) -> (.not. x?=w739:bool)
        n419 = call-poly <vilib>:"Ramp Pattern.vi"("start"=0.0, "end"=w730, "samples"=w730) -> ("Ramp Pattern"=w725:dbl[])  [unwired: 7 in, 1 out]
        n420 = call-poly <vilib>:"Ramp Pattern.vi"("start"=0.0, "end"=w729, "samples"=w729) -> ("Ramp Pattern"=w726:dbl[])  [unwired: 7 in, 1 out]
        n421 = property on="mainimg" class="IntGraph (strict)"() -> ("CrsrLis"=w718:T5)  [unwired: 2 in, 2 out]
        n422 = And(x="cam_liveavg", y=w739) -> (x .and. y?=w737:bool)
        n423 = case shown="False" w737 {
          tunnel: w736 -> [w765 w771]
          tunnel: [w765 w768] -> w713
          tunnel: w748 -> [_ w773]
          tunnel: w721 -> [w766 _]
          tunnel: [w766 w774] -> w747
          tunnel: w720 -> [_ w774]
          tunnel: w719 -> [_ w767]
          frame False {
          }
          frame True {
            n424 = Multiply(x=w773, y=w767) -> (x*y=w772:dbl[][])
            n425 = Increment(x=w767) -> (x+1=w769:i32)
            n426 = Add(x=w772, y=w771) -> (x+y=w770:dbl[][])
            n427 = Divide(x=w770, y=w769) -> (x/y=w768:dbl[][])
          }
        }
        "mainimg" <- w713
        n428 = Index Array(array=w718) -> (element #1=w716:T10, element #2=w717:T10)  [unwired: 2 in]
        n429 = Unbundle By Name(w716) -> ("Position.X"=w710:dbl, "Position.Y"=w712:dbl)
        n430 = Unbundle By Name(w717) -> ("Position.X"=w714:dbl, "Position.Y"=w715:dbl)
        n431 = Array Max & Min(array=w713) -> (max value=→"max":dbl)  [unwired: 3 out]
        n432 = Subtract(x=w715, y=w712) -> (x-y=w711:dbl)
        n433 = Subtract(x=w714, y=w710) -> (x-y=w709:dbl)
        n434 = Array Subset(array=w713, index (row)=w712, length (row)=w711) -> (w724:dbl[][])  [unwired: 2 in]
        n435 = Array Subset(array=w713, index (col)=w710, length (col)=w709) -> (w722:dbl[][])  [unwired: 2 in]
        n436 = Array Subset(array=w713, index (row)=w712, length (row)=w711, index (col)=w710, length (col)=w709) -> (w708:dbl[][])
        n437 = Transpose 2D Array(2D array=w724) -> (transposed array=w723:dbl[][])
        n438 = Add Array Elements(numeric array=w708) -> (sum=→"sum" →"Waveform Chart":dbl)
        n439 = for {
          tunnel: w722 -> [w762] mode=indexing
          tunnel: [w761] -> w732 mode=indexing
          n440 = Add Array Elements(numeric array=w762) -> (sum=w761:dbl)
        }
        n441 = for {
          tunnel: w723 -> [w764] mode=indexing
          tunnel: [w763] -> w731 mode=indexing
          n442 = Add Array Elements(numeric array=w764) -> (sum=w763:dbl)
        }
        n443 = Bundle("Ramp Pattern"=w726, w731) -> (→"G2 X":cluster{"Ramp Pattern":dbl[], dbl[]})  [unwired: 1 in]
        n444 = Bundle(w732, "Ramp Pattern"=w725) -> (→"G2 Y":cluster{dbl[], "Ramp Pattern":dbl[]})  [unwired: 1 in]
      }
      frame "dark" {
        n445 = Dequeue Element(queue=w793) -> ()  [unwired: 2 in, 4 out]
        n446 = Array Size(array=w790) -> (size(s)=w789:i32[])
        n447 = Index Array(array=w789) -> (element #1=w788:i32, element #2=w787:i32)  [unwired: 2 in]
        n448 = Initialize Array(0.0 ("element"), w788, w787) -> (w785:dbl[][])
        n449 = for {
          N: "dark avg" -> [_]
          tunnel: w795 -> [w803]
          tunnel: w794 -> [w802]
          tunnel: [w801] -> w792
          tunnel: w790 -> [w800]
          tunnel: [w799] -> w791
          shift-right: [w796] -> w783
          shift-left: w785 -> [w797]
          n450 = call "grabimg.vi"("array in"=w800, "error in"=w802, "Hin"=w803) -> ("error out"=w801:errorcluster, "imgdata"=w798:i32[][], "Hout"=w799:u64)  [unwired: 6 in]
          n451 = Add(x=w798, y=w797) -> (x+y=w796:dbl[][])
        }
        n452 = Divide(x=w783, y="dark avg") -> (x/y=w784:dbl[][])
      }
      frame "snap" {
        n453 = Dequeue Element(queue=w823) -> ()  [unwired: 2 in, 4 out]
        n454 = local read "cam_dark?"() -> (w822:bool)
        n455 = local read "cam_avgs"() -> (w817:i32)
        n456 = To Double Precision Float(number=w808) -> (double precision float=w807:dbl[][])
        n457 = Equal To 0?(x="aq.mode") -> (x = 0?=w810:bool)
        n458 = Get Date/Time In Seconds() -> (seconds since 1Jan1904=w813:timestamp)
        n459 = for {
          N: w817 -> [w835]
          shift-right: [w852] -> w818
          shift-left: w820 -> [w854]
          shift-right: [w840] -> w816
          shift-left: w819 -> [w853]
          tunnel: w822 -> [w850]
          tunnel: w821 -> [w849]
          tunnel: w808 -> [w848]
          tunnel: w813 -> [w844]
          tunnel: w810 -> [w828]
          shift-right: [w836] -> w804
          shift-left: w807 -> [w837]
          shift-right: [w826] -> w805
          shift-left: w806 -> [w826]
          i -> [w824]
          stop <- "abort acq." stop-if-true
          n460 = call "grabimg.vi"("array in"=w848, "error in"=w853, "Hin"=w854) -> ("error out"=w840:errorcluster, "imgdata"=w851:i32[][], "Hout"=w852:u64)  [unwired: 6 in]
          n461 = local read "lower threshold"() -> (w831:i32)
          n462 = Increment(x=w824) -> (x+1=w833:i32)
          "acq. imgs" <- w833
          n463 = Get Date/Time In Seconds() -> (seconds since 1Jan1904=w847:timestamp)
          n464 = case shown="True" w850 {
            tunnel: w851 -> [w876 w879]
            tunnel: w849 -> [_ w878]
            tunnel: [w876 w877] -> w830
            frame False {
            }
            frame True {
              n465 = Subtract(x=w879, y=w878) -> (x-y=w877:dbl[][])
            }
          }
          n466 = Divide(x=w833, y=w835) -> (x/y=→"snap_prog":dbl)
          n467 = Subtract(x=w847, y=w844) -> (x-y=w846:dbl)
          n468 = call "filtr_b.vi"("threshold"=w831, "input array"=w830) -> ("output array"=w829:dbl[][])  [unwired: 9 in]
          n469 = Divide(x=w846, y=w824) -> (x/y=w842:dbl)
          n470 = Multiply(x=w842, y=w835) -> (x*y=w845:dbl)
          n471 = Reciprocal(x=w842) -> (1/x=w841:dbl)
          n472 = case shown="True" "count?" {
            tunnel: w829 -> [w867 w869]
            tunnel: "e-size" -> [_ w871]
            tunnel: w831 -> [_ w870]
            tunnel: [w867 w868] -> w827
            frame False {
            }
            frame True {
              n473 = Array Size(array=w869) -> (size(s)=w873:i32[])
              n474 = call "findr.vi"("thresh"=w870, "esize"=w871, "inp array"=w869) -> ("locs"=w872:i32[][])  [unwired: 8 in]
              n475 = Index Array(array=w873) -> (element #1=w875:i32, element #2=w874:i32)  [unwired: 2 in]
              n476 = call "drawe.vi"("Ysize"=w875, "Xsize"=w874, "pos array"=w872) -> ("img out"=w868:i32[][])  [unwired: 8 in]
            }
          }
          n477 = Add(x=w845, y=w844) -> (x+y=→"ETA":timestamp)
          n478 = local write "cam_fps"(w841) -> ()
          n479 = local write "mainimg"(w829) -> ()
          n480 = case shown="True" w828 {
            tunnel: w827 -> [w857 w865]
            tunnel: w837 -> [w859 w864]
            tunnel: [w858 w862] -> w836
            tunnel: [w856 w861] -> w825
            tunnel: w824 -> [w855 w860]
            frame False {
              n481 = Add(x=w857, y=w859) -> (x+y=w858:dbl[][])
              n482 = Increment(x=w855) -> (x+1=w856:i32)
            }
            frame True {
              n483 = Multiply(x=w864, y=w860) -> (x*y=w866:dbl[][])
              n484 = Increment(x=w860) -> (x+1=w861:i32)
              n485 = Add(x=w865, y=w866) -> (x+y=w863:dbl[][])
              n486 = Divide(x=w863, y=w861) -> (x/y=w862:dbl[][])
            }
          }
          "Pics L" <- w825
          n487 = local write "sideimg"(w836) -> ()
        }
        n488 = Enqueue Element(queue=w812, element=w804, error in (no error)=w816) -> (error out=w809:errorcluster)  [unwired: 1 in, 2 out]
      }
      frame "suspend" {
        n489 = Dequeue Element(queue=w888) -> ()  [unwired: 2 in, 4 out]
      }
    }
    "cam_error" <- w606
  }
  n490 = while {
    tunnel: w4 -> [w897]
    shift-right: [w894] -> _
    shift-left: _ -> [w895]
    tunnel: w3 -> [w893]
    shift-right: [w892] -> _
    shift-left: _ -> [w891]
    shift-right: [w889] -> _
    shift-left: _ -> [w890]
    stop <- w896 stop-if-true
    # "mirr"
    n491 = Preview Queue Element(queue=w897, timeout in ms (-1)=w895) -> (queue out=w900:refnum<queue>, element=w901:string)  [unwired: 1 in, 2 out]
    n492 = Match Pattern(string=w901, regular expression=":") -> (before substring=w899:string, after substring=w898:string)  [unwired: 1 in, 2 out]
    n493 = case shown="\"abs\"" w899 {
      tunnel: w900 -> [w936 w946 w961 w965 w968 w973 _]
      tunnel: w898 -> [w930 w947 _ _ _ _ _]
      tunnel: [_ _ _ TRUE _ _ _] -> w896
      tunnel: [_ _ _ _ -1 _ _] -> w894
      tunnel: w893 -> [w903 _ _ _ _ _ _]
      tunnel: [w922 w943 refnum<visa-resource-name> refnum ("VISA resource name out") w963 w967 w972 w978] -> w892
      tunnel: w891 -> [w935 w945 w960 w963 w967 _ w982]
      tunnel: [w907 w942 w959 w962 w966 w971 w977] -> w889
      tunnel: w890 -> [w934 w944 _ w962 w966 _ w981]
      frame "abs" {
        w918 = u8 20 items=["Echo"=55, "Home"=1, "Move Absolute"=20, "Move Relative"=21, "Move at Constant Speed"=22, "Renumber"=2, "Restore Settings"=36, "Stop"=23] ("Command")
        w933 = u8 20 items=["Echo"=55, "Home"=1, "Move Absolute"=20, "Move Relative"=21, "Move at Constant Speed"=22, "Renumber"=2, "Restore Settings"=36, "Stop"=23] ("Command")
        n494 = Dequeue Element(queue=w936) -> ()  [unwired: 2 in, 4 out]
        n495 = Match Pattern(string=w930, regular expression=":") -> (before substring=w920:string, after substring=w906:string)  [unwired: 1 in, 2 out]
        n496 = Equal?(x=w906, y="confirm") -> (x = y?=w904:bool)
        n497 = Scan From String(format string="%g_%g", input string=w920) -> (output 1=w915:dbl, output 2=w914:dbl)  [unwired: 4 in, 3 out]
        n498 = local read "mirr_X#"() -> (w917:u8)
        n499 = Bundle("mirr_X#"=w917, "Command"=w933, w915, "Response Count"=1) -> (w929:T11)  [unwired: 1 in]
        n500 = local read "mirr_Y#"() -> (w916:u8)
        n501 = call "Request Command.vi"("error in (no error)"=w934, "Request"=w929, "VISA resource name"=w935) -> ("error out"=w911:errorcluster, "VISA resource name out"=w912:refnum<visa-resource-name>)  [unwired: 5 in, 2 out]
        n502 = Bundle("mirr_Y#"=w916, "Command"=w918, w914, "Response Count"=1) -> (w913:T12)  [unwired: 1 in]
        n503 = call "Request Command.vi"("error in (no error)"=w911, "Request"=w913, "VISA resource name"=w912) -> ("error out"=w909:errorcluster, "VISA resource name out"=w910:refnum<visa-resource-name>)  [unwired: 5 in, 2 out]
        n504 = local read "mirr_X#"() -> (w927:u8)
        n505 = call "zaber_readpos.vi"("error in (no error)"=w909, "axis"=w927, "VISA in"=w910) -> ("error out"=w923:errorcluster, "position"=w928:i32, "VISA out"=w924:refnum<visa-resource-name>)  [unwired: 6 in]
        n506 = local read "mirr_Y#"() -> (w925:u8)
        n507 = local write "mirr_posX"(w928) -> ()
        n508 = call "zaber_readpos.vi"("error in (no error)"=w923, "axis"=w925, "VISA in"=w924) -> ("error out"=w908:errorcluster, "position"=w926:i32, "VISA out"=w922:refnum<visa-resource-name>)  [unwired: 6 in]
        n509 = local write "mirr_posY"(w926) -> ()
        n510 = case shown="True" w904 {
          tunnel: w908 -> [w937 w941]
          tunnel: [w937 w940] -> w907
          tunnel: w903 -> [_ w939]
          frame False {
          }
          frame True {
            n511 = Send Notification(notification=TRUE, notifier=w939, error in (no error)=w941) -> (error out=w940:errorcluster)  [unwired: 1 out]
          }
        }
      }
      frame "rel" {
        w950 = u8 21 items=["Echo"=55, "Home"=1, "Move Absolute"=20, "Move Relative"=21, "Move at Constant Speed"=22, "Renumber"=2, "Restore Settings"=36, "Stop"=23] ("Command")
        n512 = Dequeue Element(queue=w946) -> ()  [unwired: 2 in, 4 out]
        n513 = Match Pattern(string=w947, regular expression=":") -> (before substring=w952:string, after substring=w951:string)  [unwired: 1 in, 2 out]
        n514 = Decimal String To Number(string=w952) -> (number=w954:i32)  [unwired: 2 in, 1 out]
        n515 = Decimal String To Number(string=w951) -> (number=w955:i32)  [unwired: 2 in, 1 out]
        n516 = Bundle(w954, "Command"=w950, w955, "Response Count"=1) -> (w948:T13)  [unwired: 1 in]
        n517 = call "Request Command.vi"("error in (no error)"=w944, "Request"=w948, "VISA resource name"=w945) -> ("error out"=w942:errorcluster, "VISA resource name out"=w943:refnum<visa-resource-name>)  [unwired: 5 in, 2 out]
      }
      frame "release" {
        n518 = Dequeue Element(queue=w961) -> (queue out=w957:refnum<queue>)  [unwired: 2 in, 3 out]
        n519 = Enqueue Element(queue=w957, element="suspend") -> ()  [unwired: 2 in, 3 out]
        n520 = call "Close.vi"("VISA resource name"=w960) -> ("error out"=w959:errorcluster)  [unwired: 9 in, 1 out]
      }
      frame "close" {
        n521 = Release Queue(queue=w965) -> ()  [unwired: 2 in, 3 out]
      }
      frame "suspend" {
        n522 = Dequeue Element(queue=w968) -> ()  [unwired: 2 in, 4 out]
      }
      frame "init" {
        n523 = Dequeue Element(queue=w973) -> ()  [unwired: 2 in, 4 out]
        n524 = call "Initialize.vi"("VISA resource name"="mirr_VISA") -> ("error out"=w971:errorcluster, "VISA resource name out"=w972:refnum<visa-resource-name>)  [unwired: 8 in, 1 out]
      }
      frame "idle", Default {
        n525 = local read "mirr_X#"() -> (w983:u8)
        n526 = call "zaber_readpos.vi"("error in (no error)"=w981, "axis"=w983, "VISA in"=w982) -> ("error out"=w979:errorcluster, "position"=→"mirr_posX":i32, "VISA out"=w980:refnum<visa-resource-name>)  [unwired: 6 in]
        n527 = local read "mirr_Y#"() -> (w976:u8)
        n528 = call "zaber_readpos.vi"("error in (no error)"=w979, "axis"=w976, "VISA in"=w980) -> ("error out"=w977:errorcluster, "position"=→"mirr_posY":i32, "VISA out"=w978:refnum<visa-resource-name>)  [unwired: 6 in]
      }
    }
    "mirr_Error" <- w889
  }
  n529 = while {
    tunnel: w13 -> [w992]
    shift-right: [w990] -> _
    shift-left: _ -> [w988]
    shift-right: [w989] -> _
    shift-left: _ -> [w987]
    shift-right: [w985] -> _
    shift-left: 0 -> [w986]
    tunnel: w3 -> [w984]
    stop <- w991 stop-if-true
    # "ESP"
    n530 = Preview Queue Element(queue=w992, timeout in ms (-1)=w986) -> (queue out=w995:refnum<queue>, element=w996:string)  [unwired: 1 in, 2 out]
    n531 = Match Pattern(string=w996, regular expression=":") -> (before substring=w994:string, after substring=w993:string)  [unwired: 1 in, 2 out]
    n532 = case shown="\"abs\"" w994 {
      tunnel: w995 -> [_ w1007 w1025 w1066 w1069 w1076 w1081]
      tunnel: w993 -> [_ w1012 w1032 _ _ _ _]
      tunnel: [_ _ _ _ _ TRUE _] -> w991
      tunnel: [w999 w1014 w1026 w1064 refnum<visa-resource-name> refnum ("VISA resource name out") w1073 w1080] -> w990
      tunnel: [w998 w1015 w1024 w1063 w1071 w1074 w1079] -> w989
      tunnel: w988 -> [w1003 w1017 w1030 w1064 w1072 w1073 _]
      tunnel: w987 -> [w1002 w1016 w1031 w1063 _ w1074 _]
      tunnel: [_ _ _ -1 _ _ _] -> w985
      tunnel: w984 -> [_ _ w1018 _ _ _ _]
      frame "idle", Default {
        n533 = local read "ESP Axis"() -> (w1000:i32)
        n534 = local read "ESP_t0"() -> (w1006:dbl)
        n535 = call "Read Actual Position.vi"("error in (no error)"=w1002, "Axis (1)"=w1000, "VISA resource name"=w1003) -> ("error out"=w998:errorcluster, "Position (units)"=w1001:dbl, "VISA resource name out"=w999:refnum<visa-resource-name>)  [unwired: 2 in]
        "ESP_pos" <- w1001
        n536 = call "mm2time.vi"("fs?"=TRUE, "Offset (mm)"=w1006, "distance (mm)"=w1001) -> ("time in fs/ps seconds"=→"ESP_delay":dbl)
      }
      frame "rel" {
        n537 = Match Pattern(string=w1012, regular expression=":") -> (before substring=w1011:string, after substring=w1010:string)  [unwired: 1 in, 2 out]
        n538 = Dequeue Element(queue=w1007) -> ()  [unwired: 2 in, 4 out]
        n539 = Decimal String To Number(string=w1011) -> (number=w1009:i32)  [unwired: 2 in, 1 out]
        n540 = Fract/Exp String To Number(string=w1010) -> (number=w1008:dbl)  [unwired: 3 in, 1 out]
        n541 = call "Move Relative.vi"("error in (no error)"=w1016, "Position (0 units)"=w1008, "Axis (1)"=w1009, "VISA resource name"=w1017) -> ("error out"=w1015:errorcluster, "VISA resource name out"=w1014:refnum<visa-resource-name>)  [unwired: 2 in]
      }
      frame "abs" {
        n542 = Dequeue Element(queue=w1025) -> ()  [unwired: 2 in, 4 out]
        n543 = Match Pattern(string=w1032, regular expression=":") -> (before substring=w1033:string, after substring=w1022:string)  [unwired: 1 in, 2 out]
        n544 = Match Pattern(string=w1022, regular expression=":") -> (before substring=w1021:string, after substring=w1020:string)  [unwired: 1 in, 2 out]
        n545 = Decimal String To Number(string=w1033) -> (number=w1029:i32)  [unwired: 2 in, 1 out]
        n546 = Fract/Exp String To Number(string=w1021) -> (number=w1019:dbl)  [unwired: 3 in, 1 out]
        n547 = call "Move Absolute.vi"("error in (no error)"=w1031, "Position (0 units)"=w1019, "Axis (1)"=w1029, "VISA resource name"=w1030) -> ("error out"=w1027:errorcluster, "VISA resource name out"=w1028:refnum<visa-resource-name>)  [unwired: 2 in]
        n548 = case shown="\"confirm\"" w1020 {
          tunnel: w1029 -> [_ w1051]
          tunnel: w1028 -> [w1036 w1053]
          tunnel: w1027 -> [w1035 w1052]
          tunnel: [w1036 w1039] -> w1026
          tunnel: [w1035 w1048] -> w1024
          tunnel: w1018 -> [_ w1047]
          frame "", Default {
          }
          frame "confirm" {
            n549 = while {
              tunnel: w1051 -> [w1062]
              shift-right: [w1059] -> w1050
              shift-left: w1053 -> [w1061]
              shift-right: [w1058] -> w1049
              shift-left: w1052 -> [w1060]
              stop <- w1057 stop-if-true
              n550 = call "Get Axis Motion Status.vi"("error in (no error)"=w1060, "Axis (1)"=w1062, "VISA resource name"=w1061) -> ("error out"=w1058:errorcluster, "Motion Done"=w1057:bool, "VISA resource name out"=w1059:refnum<visa-resource-name>)  [unwired: 2 in]
            }
            n551 = flat-sequence {
              tunnel: w1050 -> [w1056]
              tunnel: w1049 -> [w1055]
              tunnel: [w1056] -> w1042
              tunnel: [w1055] -> w1041
              frame #0 {
                n552 = Wait (ms)(milliseconds to wait=u32 1000) -> ()  [unwired: 1 out]
              }
            }
            n553 = local read "ESP Axis"() -> (w1043:i32)
            n554 = local read "ESP_t0"() -> (w1045:dbl)
            n555 = call "Read Actual Position.vi"("error in (no error)"=w1041, "Axis (1)"=w1043, "VISA resource name"=w1042) -> ("error out"=w1040:errorcluster, "Position (units)"=w1037:dbl, "VISA resource name out"=w1039:refnum<visa-resource-name>)  [unwired: 2 in]
            n556 = call "mm2time.vi"("fs?"=TRUE, "Offset (mm)"=w1045, "distance (mm)"=w1037) -> ("time in fs/ps seconds"=w1038:dbl)
            n557 = local write "ESP_pos"(w1037) -> ()
            n558 = local write "ESP_delay"(w1038) -> ()
            n559 = Send Notification(notification=TRUE, notifier=w1047, error in (no error)=w1040) -> (error out=w1048:errorcluster)  [unwired: 1 out]
          }
        }
      }
      frame "suspend" {
        n560 = Dequeue Element(queue=w1066) -> ()  [unwired: 2 in, 4 out]
      }
      frame "release" {
        n561 = Dequeue Element(queue=w1069) -> (queue out=w1067:refnum<queue>)  [unwired: 2 in, 3 out]
        n562 = call "Close.vi"("VISA resource name"=w1072) -> ("error out"=w1071:errorcluster)  [unwired: 10 in]
        n563 = Enqueue Element(queue=w1067, element="suspend") -> ()  [unwired: 2 in, 3 out]
      }
      frame "close" {
        n564 = Release Queue(queue=w1076) -> ()  [unwired: 2 in, 3 out]
      }
      frame "init" {
        n565 = Dequeue Element(queue=w1081) -> ()  [unwired: 2 in, 4 out]
        n566 = flat-sequence {
          tunnel: [w1084] -> w1078
          tunnel: [w1083] -> w1077
          tunnel: [w1088] -> w1079
          tunnel: [w1089] -> w1080
          tunnel: w1078 -> [w1089]
          tunnel: w1077 -> [w1088]
          frame #0 {
            n567 = local write "ESP_con?"(FALSE ("ESP_con?")) -> ()
          }
          frame #1 {
            n568 = call "Initialize.vi"("VISA resource name"="ESP301 VISA", "Serial Link (RS232)"=enum16{"RS232", "USB"}."USB") -> ("VISA resource name out"=w1084:refnum<visa-resource-name>, "error out"=w1083:errorcluster)  [unwired: 7 in]
          }
          frame #2 {
            n569 = local write "ESP_con?"(TRUE ("ESP_con?")) -> ()
          }
        }
      }
    }
    "error out" <- w989
  }
  n570 = while {
    tunnel: w12 -> [w1098]
    shift-right: [w1096] -> _
    shift-left: _ -> [w1094]
    shift-right: [w1095] -> _
    shift-left: _ -> [w1093]
    shift-right: [w1091] -> _
    shift-left: 0 -> [w1092]
    tunnel: w3 -> [w1090]
    stop <- w1097 stop-if-true
    # "manip"
    n571 = Preview Queue Element(queue=w1098, timeout in ms (-1)=w1092) -> (queue out=w1101:refnum<queue>, element=w1102:string)  [unwired: 1 in, 2 out]
    n572 = Match Pattern(string=w1102, regular expression=":") -> (before substring=w1100:string, after substring=w1099:string)  [unwired: 1 in, 2 out]
    n573 = case shown="\"rel\"" w1100 {
      tunnel: w1101 -> [_ w1114 w1141 w1182 w1220 w1226 w1235 w1240]
      tunnel: w1099 -> [_ _ w1128 w1181 _ _ _ _]
      tunnel: [_ _ _ _ _ _ TRUE _] -> w1097
      tunnel: [w1108 w1116 w1120 w1179 w1222 refnum<k5> refnum ("gateway_connection out") w1233 w1239] -> w1096
      tunnel: [w1107 w1115 w1122 w1178 w1221 w1228 w1232 w1238] -> w1095
      tunnel: w1094 -> [w1110 w1118 w1144 w1172 w1222 w1230 w1233 _]
      tunnel: w1093 -> [w1109 w1117 w1143 w1173 w1221 _ w1232 _]
      tunnel: [_ _ _ _ -1 _ _ _] -> w1091
      tunnel: w1090 -> [_ _ w1119 w1175 _ _ _ _]
      frame "idle", Default {
        n574 = call "sp_manip_get_axis_status.vi"("error in"=w1109, "gateway_connection"=w1110) -> ("error out"=w1107:errorcluster, "axis_out"=w1106:T14, "gateway_connection out"=w1108:refnum<k5>)  [unwired: 5 in, 2 out]
        n575 = for {
          tunnel: w1106 -> [w1113] mode=indexing
          tunnel: [w1112] -> w1105 mode=indexing
          tunnel: [w1111] -> w1104 mode=indexing
          n576 = Unbundle By Name(w1113) -> ("Axis_Position"=w1112:dbl, "moving"=w1111:bool)
        }
        "moving?" <- w1104
        n577 = local write "pos"(w1105) -> ()
      }
      frame "stop" {
        n578 = Dequeue Element(queue=w1114) -> ()  [unwired: 2 in, 4 out]
        n579 = call "sp_manip_abort.vi"("error in"=w1117, "gateway_connection"=w1118) -> ("error out"=w1115:errorcluster, "gateway_connection out"=w1116:refnum<k5>)  [unwired: 6 in, 2 out]
      }
      frame "rel" {
        n580 = Dequeue Element(queue=w1141) -> ()  [unwired: 2 in, 4 out]
        n581 = Match Pattern(string=w1128, regular expression=":") -> (before substring=w1127:string, after substring=w1126:string)  [unwired: 1 in, 2 out]
        n582 = Equal?(x=w1126, y="confirm") -> (x = y?=w1124:bool)
        n583 = call "sp_manip_get_axis_status.vi"("error in"=w1143, "gateway_connection"=w1144) -> ("error out"=w1146:errorcluster, "axis_out"=w1133:T14, "gateway_connection out"=w1145:refnum<k5>)  [unwired: 5 in, 2 out]
        n584 = Scan From String(format string="%g_%g_%g_%g_%g_%g", input string=w1127) -> (output 1=w1140:dbl, output 2=w1139:dbl, output 3=w1138:dbl, output 4=w1137:dbl, output 5=w1136:dbl, output 6=w1135:dbl)  [unwired: 8 in, 3 out]
        n585 = for {
          tunnel: w1133 -> [w1167] mode=indexing
          tunnel: [w1166] -> w1131 mode=indexing
          tunnel: [w1165] -> w1132 mode=indexing
          n586 = Unbundle By Name(w1167) -> ("Axis_Name"=w1166:string, "Axis_Position"=w1165:dbl)
        }
        n587 = Build Array(w1140, w1139, w1138, w1137, w1136, w1135) -> (w1134:dbl[])
        n588 = Add(x=w1132, y=w1134) -> (x+y=w1130:dbl[])
        n589 = call "sp_manip_start_move.vi"("error in"=w1146, "target positions"=w1130, "axis names"=w1131, "gateway_connection"=w1145) -> ("error out"=w1123:errorcluster, "gateway_connection out"=w1121:refnum<k5>)  [unwired: 4 in, 2 out]
        n590 = case shown="True" w1124 {
          tunnel: w1123 -> [w1147 w1154]
          tunnel: [w1147 w1151] -> w1122
          tunnel: w1121 -> [w1148 w1155]
          tunnel: [w1148 w1153] -> w1120
          tunnel: w1119 -> [_ w1150]
          frame False {
          }
          frame True {
            n591 = while {
              tunnel: w1155 -> [w1159]
              tunnel: w1154 -> [w1158]
              tunnel: [w1157] -> w1153
              tunnel: [w1156] -> w1152
              stop <- w1160 continue-if-true
              n592 = call "sp_manip_get_axis_status.vi"("error in"=w1158, "gateway_connection"=w1159) -> ("error out"=w1156:errorcluster, "axis_out"=w1162:T14, "gateway_connection out"=w1157:refnum<k5>)  [unwired: 5 in, 2 out]
              n593 = for {
                tunnel: w1162 -> [w1164] mode=indexing
                tunnel: [w1163] -> w1161 mode=indexing
                n594 = Unbundle By Name(w1164) -> ("moving"=w1163:bool)
              }
              n595 = Or Array Elements(Boolean array=w1161) -> (logical OR=w1160:bool)
            }
            n596 = Send Notification(notification=TRUE, notifier=w1150, error in (no error)=w1152) -> (error out=w1151:errorcluster)  [unwired: 1 out]
          }
        }
      }
      frame "abs" {
        n597 = Dequeue Element(queue=w1182) -> ()  [unwired: 2 in, 4 out]
        n598 = call "sp_manip_get_axis_status.vi"("error in"=w1173, "gateway_connection"=w1172) -> ("error out"=w1168:errorcluster, "axis_out"=w1171:T14, "gateway_connection out"=w1169:refnum<k5>)  [unwired: 5 in, 2 out]
        n599 = Match Pattern(string=w1181, regular expression=":") -> (before substring=w1185:string, after substring=w1184:string)  [unwired: 1 in, 2 out]
        n600 = Equal?(x=w1184, y="wait") -> (x = y?=w1174:bool)
        n601 = for {
          tunnel: w1171 -> [w1195] mode=indexing
          tunnel: [w1194] -> w1170 mode=indexing
          n602 = Unbundle By Name(w1195) -> ("Axis_Name"=w1194:string)
        }
        n603 = Scan From String(format string="%g_%g_%g_%g_%g_%g", input string=w1185) -> (output 1=w1191:dbl, output 2=w1190:dbl, output 3=w1189:dbl, output 4=w1188:dbl, output 5=w1187:dbl, output 6=w1186:dbl)  [unwired: 8 in, 3 out]
        n604 = Build Array(w1191, w1190, w1189, w1188, w1187, w1186) -> (w1193:dbl[])
        n605 = call "sp_manip_start_move.vi"("error in"=w1168, "target positions"=w1193, "axis names"=w1170, "gateway_connection"=w1169) -> ("error out"=w1177:errorcluster, "gateway_connection out"=w1176:refnum<k5>)  [unwired: 4 in, 2 out]
        n606 = case shown="True" w1174 {
          tunnel: w1177 -> [w1196 w1207]
          tunnel: [w1196 w1206] -> w1178
          tunnel: w1176 -> [w1197 w1208]
          tunnel: [w1197 w1199] -> w1179
          tunnel: w1175 -> [_ w1205]
          frame False {
          }
          frame True {
            n607 = while {
              tunnel: w1208 -> [w1214]
              tunnel: w1207 -> [w1213]
              tunnel: [w1212] -> w1201
              tunnel: [w1211] -> w1200
              stop <- w1215 continue-if-true
              n608 = call "sp_manip_get_axis_status.vi"("error in"=w1213, "gateway_connection"=w1214) -> ("error out"=w1211:errorcluster, "axis_out"=w1217:T14, "gateway_connection out"=w1212:refnum<k5>)  [unwired: 5 in, 2 out]
              n609 = for {
                tunnel: w1217 -> [w1219] mode=indexing
                tunnel: [w1218] -> w1216 mode=indexing
                n610 = Unbundle By Name(w1219) -> ("moving"=w1218:bool)
              }
              n611 = Or Array Elements(Boolean array=w1216) -> (logical OR=w1215:bool)
            }
            n612 = call "sp_manip_get_axis_status.vi"("error in"=w1200, "gateway_connection"=w1201) -> ("error out"=w1198:errorcluster, "axis_out"=w1203:T14, "gateway_connection out"=w1199:refnum<k5>)  [unwired: 5 in, 2 out]
            n613 = for {
              tunnel: w1203 -> [w1210] mode=indexing
              tunnel: [w1209] -> w1202 mode=indexing
              n614 = Unbundle By Name(w1210) -> ("Axis_Position"=w1209:dbl)
            }
            n615 = local write "pos"(w1202) -> ()
            n616 = Send Notification(notification=TRUE, notifier=w1205, error in (no error)=w1198) -> (error out=w1206:errorcluster)  [unwired: 1 out]
          }
        }
      }
      frame "suspend" {
        n617 = Dequeue Element(queue=w1220) -> ()  [unwired: 2 in, 4 out]
      }
      frame "release" {
        n618 = Dequeue Element(queue=w1226) -> (queue out=w1224:refnum<queue>)  [unwired: 2 in, 3 out]
        n619 = call "sp_manip_disconnect.vi"("gateway_connection"=w1230) -> ("error out"=w1229:errorcluster, "gateway_connection_out"=w1231:refnum<k5>)  [unwired: 7 in, 2 out]
        n620 = call "tcp_gateway_close_connection.vi"("error in"=w1229, "server_connection"=w1231) -> ("error out"=w1228:errorcluster)  [unwired: 5 in]
        n621 = Enqueue Element(queue=w1224, element="suspend") -> ()  [unwired: 2 in, 3 out]
      }
      frame "close" {
        n622 = Release Queue(queue=w1235) -> ()  [unwired: 2 in, 3 out]
      }
      frame "init" {
        n623 = Dequeue Element(queue=w1240) -> ()  [unwired: 2 in, 4 out]
        n624 = flat-sequence {
          tunnel: [w1243] -> w1237
          tunnel: [w1242] -> w1236
          tunnel: [w1253] -> w1238
          tunnel: [w1254] -> w1239
          tunnel: w1237 -> [w1254]
          tunnel: w1236 -> [w1253]
          frame #0 {
            n625 = local write "manip_con?"(FALSE ("manip_con?")) -> ()
          }
          frame #1 {
            n626 = call "tcp_gateway_open_connection.vi"() -> ("gateway_connection"=w1246:refnum<k5>, "error out"=w1245:errorcluster)  [unwired: 5 in, 3 out]
            n627 = call "sp_manip_connect.vi"("error in"=w1245, "gateway_connection"=w1246) -> ("error out"=w1242:errorcluster, "axis_out"=w1244:T14, "gateway_connection out"=w1243:refnum<k5>)  [unwired: 5 in, 2 out]
            n628 = for {
              tunnel: w1244 -> [w1251] mode=indexing
              tunnel: [w1250] -> w1247 mode=indexing
              tunnel: [w1249] -> w1248 mode=indexing
              n629 = Unbundle By Name(w1251) -> ("Axis_Name"=w1250:string, "Axis_Position"=w1249:dbl)
            }
            "axis" <- w1247
            "pos" <- w1248
            n630 = local write "dest"(w1248) -> ()
          }
          frame #2 {
            n631 = local write "manip_con?"(TRUE ("manip_con?")) -> ()
          }
        }
      }
    }
    "error out 2" <- w1095
  }
  n632 = while {
    tunnel: w11 -> [w1266]
    shift-right: [w1255] -> _
    shift-left: 0 -> [w1264]
    shift-right: [w1263] -> _
    shift-left: _ -> [w1262]
    shift-right: [w1261] -> _
    shift-left: _ -> [w1260]
    shift-right: [w1259] -> _
    shift-left: u32 0 ("pHandle") -> [w1258]
    tunnel: w9 -> [w1257]
    tunnel: w3 -> [w1256]
    stop <- w1265 stop-if-true
    # "phoib"
    n633 = Preview Queue Element(queue=w1266, timeout in ms (-1)=w1264) -> (queue out=w1269:refnum<queue>, element=w1270:string)  [unwired: 1 in, 2 out]
    n634 = Match Pattern(string=w1270, regular expression=":") -> (before substring=w1268:string, after substring=w1267:string)  [unwired: 1 in, 2 out]
    n635 = case shown="\"idle\", Default" w1268 {
      tunnel: w1269 -> [_ w1323 w1377 w1394 w1412 w1426 w1431 w1436]
      tunnel: w1267 -> [_ _ w1373 _ _ _ _ _]
      tunnel: [_ _ _ _ _ TRUE _ _] -> w1265
      tunnel: [w1280 w1325 w1342 w1397 w1410 w1424 w1430 w1433] -> w1263
      tunnel: w1262 -> [w1291 w1314 w1363 w1399 w1411 w1424 w1430 _]
      tunnel: [w1279 w1324 w1358 w1396 w1409 w1422 w1428 w1432] -> w1261
      tunnel: w1260 -> [w1289 w1313 _ w1398 _ w1422 w1428 _]
      tunnel: [w1277 w1311 w1341 w1395 w1408 w1423 w1429 w1435] -> w1259
      tunnel: w1258 -> [w1277 w1311 w1361 w1395 w1407 w1423 w1429 _]
      tunnel: w1257 -> [w1278 w1304 w1339 _ _ _ _ _]
      tunnel: w1256 -> [_ _ w1357 _ _ _ _ _]
      tunnel: [_ _ _ _ _ _ -1 _] -> w1255
      frame "idle", Default {
        n636 = call "SL2_AD_DLL_Phoibos_GetDeviceState.vi"("dll_path"=w1291, "pHandle_in"=w1277, "dev_type"=DEF_dev_type."devA (analyzer)", "error in"=w1289) -> ("path out"=w1276:path, "state"=→"state":T3, "error out"=w1275:errorcluster)  [unwired: 2 in]
        n637 = for {
          tunnel: w1277 -> [w1298]
          tunnel: w1278 -> [w1296] mode=indexing
          tunnel: [w1295] -> w1288 mode=indexing
          tunnel: [w1294] -> w1280
          shift-right: [w1293] -> w1279
          shift-left: w1275 -> [w1297]
          tunnel: w1276 -> [w1292]
          n638 = call "SL2_AD_DLL_Phoibos_GetVoltage.vi"("error in"=w1297, "voltage_name"=w1296, "pHandle"=w1298, "dll path in"=w1292) -> ("error out"=w1293:errorcluster, "value"=w1295:dbl, "dll path out"=w1294:path)  [unwired: 3 in]
        }
        n639 = Index Array(array=w1288) -> (element #1=→"phoib_I_1":dbl, element #2=→"phoib_I_2":dbl, element #3=→"phoib_I_3":dbl, element #4=→"phoib_I_4":dbl, element #5=→"phoib_I_5":dbl, element #6=→"phoib_I_6":dbl, element #7=→"phoib_I_7":dbl, element #8=→"phoib_I_8":dbl, element #9=→"phoib_I_9":dbl)  [unwired: 9 in]
      }
      frame "set" {
        n640 = Dequeue Element(queue=w1323) -> ()  [unwired: 2 in, 4 out]
        n641 = Multiply(x="ana_voltrange", y=13) -> (x*y=w1320:i32)
        n642 = Add(x="ana_mode", y=w1320) -> (x+y=w1317:i32)
        n643 = Index Array(array=u32[] [251749632, 251749633, 251749634, 251749635, 251749636, 251749637, 251749638, 251749639, 251749640, 251749641, 251749642, 251749643, 251749644, 251749645, 251749646, 251749647, 251749648, 251749649, 251749650, 251749651, 251749652, 251749653, 251749654, 251749655, 251749656, 251749657, 251749658, 251749659, 251749660, 251749661, 251749662, 251749663, 251749664, 251749665, 251749666, 251749667, 251749668, 251749669, 251749670, 251749671, 251749672, 251749673, 251749674, 251749675, 251749676, 251749677, 251749678, 251749679, 251749680, 251749681, 251749682, 251749683, 251749684, 251749685, 251749686, 251749687, 251749688, 251749689, 251749690, 251749691, 251749692, 251749693, 251749694, 251749695, 251749696] ("modeIDs"), index=w1317) -> (element=w1315:u32)
        n644 = Build Array("phoib_I_1s", "phoib_I_2s", "phoib_I_3s", "phoib_I_4s", "phoib_I_5s", "phoib_I_6s", "phoib_I_7s", "phoib_I_8s", "phoib_I_9s") -> (w1303:dbl[])
        n645 = call "SL2_AD_DLL_Phoibos_SetDeviceMode.vi"("pHandle"=w1311, "error in"=w1313, "value"=w1315, "dev_type"=DEF_dev_type."devA (analyzer)", "dll path in"=w1314) -> ("error out"=w1302:errorcluster, "dll path out"=w1312:path)  [unwired: 4 in]
        n646 = for {
          tunnel: w1311 -> [w1331]
          shift-right: [w1338] -> w1325
          shift-left: w1312 -> [w1335]
          tunnel: w1304 -> [w1330] mode=indexing
          tunnel: w1303 -> [w1329] mode=indexing
          shift-right: [w1337] -> w1324
          shift-left: w1302 -> [w1333]
          n647 = call "SL2_AD_DLL_Phoibos_GetVoltageRange.vi"("error in"=w1333, "voltage_name"=w1330, "pHandle"=w1331, "dll path in"=w1335) -> ("error out"=w1332:errorcluster, "min"=w1327:dbl, "max"=w1328:dbl, "dll path out"=w1334:path)  [unwired: 2 in]
          n648 = In Range and Coerce(upper limit=w1328, x=w1329, lower limit=w1327) -> (coerced(x)=w1326:dbl)  [unwired: 1 out]
          n649 = call "SL2_AD_DLL_Phoibos_SetVoltage.vi"("commit"=TRUE, "pHandle"=w1331, "error in"=w1332, "value"=w1326, "voltageName"=w1330, "dll path in"=w1334) -> ("error out"=w1337:errorcluster, "dll path out"=w1338:path)  [unwired: 3 in]
        }
      }
      frame "setsgl" {
        n650 = Dequeue Element(queue=w1377) -> ()  [unwired: 2 in, 4 out]
        n651 = Match Pattern(string=w1373, regular expression=":") -> (before substring=w1366:string, after substring=w1375:string)  [unwired: 1 in, 2 out]
        n652 = Equal?(x=w1375, y="wait") -> ()  [unwired: 1 out]
        n653 = Match Pattern(string=w1366, regular expression=":") -> (before substring=w1340:string, after substring=w1365:string)  [unwired: 1 in, 2 out]
        n654 = Fract/Exp String To Number(string=w1365) -> (number=w1364:dbl)  [unwired: 3 in, 1 out]
        n655 = call "SL2_AD_DLL_Phoibos_GetVoltageRange.vi"("voltage_name"=w1340, "pHandle"=w1361, "dll path in"=w1363) -> ("error out"=w1370:errorcluster, "min"=w1368:dbl, "max"=w1369:dbl, "dll path out"=w1371:path)  [unwired: 3 in]
        n656 = In Range and Coerce(upper limit=w1369, x=w1364, lower limit=w1368) -> (coerced(x)=w1359:dbl)  [unwired: 1 out]
        n657 = call "SL2_AD_DLL_Phoibos_SetVoltage.vi"("commit"=TRUE, "pHandle"=w1361, "error in"=w1370, "value"=w1359, "voltageName"=w1340, "dll path in"=w1371) -> ("error out"=w1360:errorcluster, "dll path out"=w1362:path)  [unwired: 3 in]
        n658 = while {
          tunnel: w1362 -> [w1393]
          tunnel: w1361 -> [w1387]
          tunnel: w1340 -> [w1392]
          tunnel: w1360 -> [w1391]
          tunnel: w1359 -> [w1390]
          tunnel: [w1387] -> w1341
          tunnel: [w1386] -> w1343
          tunnel: [w1385] -> w1345
          stop <- w1388 stop-if-true
          n659 = call "SL2_AD_DLL_Phoibos_GetVoltage.vi"("error in"=w1391, "voltage_name"=w1392, "pHandle"=w1387, "dll path in"=w1393) -> ("error out"=w1385:errorcluster, "value"=w1389:dbl, "dll path out"=w1386:path)  [unwired: 3 in]
          n660 = Equal?(x=w1390, y=w1389) -> (x = y?=w1388:bool)
        }
        n661 = for {
          tunnel: w1341 -> [w1384]
          tunnel: [w1382] -> w1346 mode=indexing
          tunnel: [w1381] -> w1342
          shift-right: [w1380] -> w1344
          shift-left: w1345 -> [w1383]
          tunnel: w1343 -> [w1379]
          tunnel: w1339 -> [w1378] mode=indexing
          n662 = call "SL2_AD_DLL_Phoibos_GetVoltage.vi"("error in"=w1383, "voltage_name"=w1378, "pHandle"=w1384, "dll path in"=w1379) -> ("error out"=w1380:errorcluster, "value"=w1382:dbl, "dll path out"=w1381:path)  [unwired: 3 in]
        }
        n663 = Index Array(array=w1346) -> (element #1=w1347:dbl, element #2=w1348:dbl, element #3=w1349:dbl, element #4=w1350:dbl, element #5=w1351:dbl, element #6=w1355:dbl, element #7=w1352:dbl, element #8=w1353:dbl, element #9=w1354:dbl)  [unwired: 9 in]
        n664 = local write "phoib_I_1"(w1347) -> ()
        n665 = local write "phoib_I_2"(w1348) -> ()
        n666 = local write "phoib_I_3"(w1349) -> ()
        n667 = local write "phoib_I_4"(w1350) -> ()
        n668 = local write "phoib_I_5"(w1351) -> ()
        n669 = local write "phoib_I_6"(w1355) -> ()
        n670 = local write "phoib_I_7"(w1352) -> ()
        n671 = local write "phoib_I_8"(w1353) -> ()
        n672 = local write "phoib_I_9"(w1354) -> ()
        n673 = Send Notification(notification=TRUE, notifier=w1357, error in (no error)=w1344) -> (error out=w1358:errorcluster)  [unwired: 1 out]
      }
      frame "standby" {
        w1400 = T3 0 items=["Off"=-1, "Standby"=0, "On"=1] ("state")
        n674 = Dequeue Element(queue=w1394) -> ()  [unwired: 2 in, 4 out]
        n675 = call "SL2_AD_DLL_Phoibos_SetDeviceState.vi"("pHandle_in"=w1395, "error in"=w1398, "state"=w1400, "dev_type"=DEF_dev_type."devA (analyzer)", "dll_path"=w1399) -> ("error out"=w1396:errorcluster, "path out"=w1397:path)  [unwired: 2 in]
      }
      frame "release" {
        n676 = Dequeue Element(queue=w1412) -> (queue out=w1402:refnum<queue>)  [unwired: 2 in, 3 out]
        n677 = flat-sequence {
          tunnel: w1411 -> [w1413]
          tunnel: w1407 -> [w1414]
          tunnel: [w1417] -> w1406
          tunnel: [w1416] -> w1405
          tunnel: [u32 0] -> w1404
          tunnel: [w1419] -> w1408
          tunnel: [w1420] -> w1409
          tunnel: [w1421] -> w1410
          tunnel: w1406 -> [w1421]
          tunnel: w1405 -> [w1420]
          tunnel: w1404 -> [w1419]
          frame #0 {
            n678 = call "SL2_AD_DLL_Phoibos_Shutdown.vi"("pHandle"=w1414, "dll path in"=w1413) -> ("error out"=w1416:errorcluster, "dll path out"=w1417:path)  [unwired: 4 in]
          }
          frame #1 {
            n679 = local write "phoib_con?"(FALSE ("phoib_con?")) -> ()
          }
        }
        n680 = Enqueue Element(queue=w1402, element="suspend") -> ()  [unwired: 2 in, 3 out]
      }
      frame "close" {
        n681 = Release Queue(queue=w1426) -> ()  [unwired: 2 in, 3 out]
      }
      frame "suspend" {
        n682 = Dequeue Element(queue=w1431) -> ()  [unwired: 2 in, 4 out]
      }
      frame "init" {
        n683 = Dequeue Element(queue=w1436) -> ()  [unwired: 2 in, 4 out]
        n684 = flat-sequence {
          tunnel: [w1443] -> w1434
          tunnel: [w1439] -> w1433
          tunnel: [w1438] -> w1432
          tunnel: [w1451] -> w1435
          tunnel: w1434 -> [w1451]
          frame #0 {
            n685 = local write "phoib_con?"(FALSE ("phoib_con?")) -> ()
          }
          frame #1 {
            w1442 = DEF_dev_type."devA (analyzer)" ("dev_type")
            n686 = call "GetSL2AD_VI_dllPath.vi"() -> ("error"=w1446:errorcluster, "Path"=w1447:path)  [unwired: 9 in, 1 out]
            n687 = call "SL2_AD_DLL_List_Devices.vi"("error in"=w1446, "dev_type"=w1442, "dll path in"=w1447) -> ("error out"=w1440:errorcluster, "devices"=w1449:string[], "dll path out"=w1441:path)  [unwired: 2 in]
            n688 = Index Array(array=w1449) -> (element=w1448:string)  [unwired: 1 in]
            n689 = call "SL2_AD_DLL_Phoibos_Initialize.vi"("error in"=w1440, "analyzerId"=w1448, "dll_path"=w1441) -> ("error out"=w1444:errorcluster, "pHandle"=w1443:u32, "path out"=w1445:path)  [unwired: 2 in]
            n690 = call "SL2_AD_DLL_Phoibos_ListDeviceModes.vi"("dll path in"=w1445, "dev_type"=w1442, "pHandle"=w1443, "error in"=w1444) -> ("dll path out"=w1439:path, "error out"=w1438:errorcluster)  [unwired: 1 in, 2 out]
          }
          frame #2 {
            n691 = local write "phoib_con?"(TRUE ("phoib_con?")) -> ()
          }
        }
      }
    }
    "phoib_error" <- w1261
  }
